vi "FL24 Washer Tool Main.vi"() -> ()   [LabVIEW 2016]
uses:
  Common/LabVIEW GEA2 Toolkit/LabVIEW_GEA2_Toolkit.lvlibp/type defs/Data In.ctl
  Common/LabVIEW GEA2 Toolkit/LabVIEW_GEA2_Toolkit.lvlibp/type defs/Source_Destination.ctl
  Common/LabVIEW GEA2 Toolkit/LabVIEW_GEA2_Toolkit.lvlibp/type defs/Data Type.ctl
  Common/LabVIEW GEA2 Toolkit/LabVIEW_GEA2_Toolkit.lvlibp/type defs/ERD Read Data In.ctl
  Laundry Tool 2.0 Support/type defs2/Select _Graph_Brass.ctl
  Laundry Tool 1.0 Support/type defs/ERD_Graph_All.ctl
  Laundry Tool 1.0 Support/type defs/ERD_Graph.ctl
  Laundry Tool 1.0 Support/type defs/Version.ctl
  Laundry Tool 2.0 Support/type defs2/ERD_Always_Show_Brass.ctl
  Laundry Tool 1.0 Support/type defs/Fault_Buffer_Status.ctl
  Laundry Tool 2.0 Support/type defs2/Diagnostics_Table.ctl
  Laundry Tool 1.0 Support/type defs/Cycle_Diag_Buffer_Status.ctl
  Laundry Tool 1.0 Support/type defs/Motor Control.ctl
  Laundry Tool 1.0 Support/type defs/Valves.ctl
  Laundry Tool 2.0 Support/type defs2/Programming_Brass.ctl
  Laundry Tool 2.0 Support/type defs2/Flash_Results.ctl
  Laundry Tool 2.0 Support/type defs2/ERD_Data_Loop_Control_Brass.ctl
  Laundry Tool 2.0 Support/type defs2/ERD_Loop_States_Brass.ctl
  Laundry Tool 2.0 Support/type defs2/Error_Command_Brass.ctl
  Laundry Tool 2.0 Support/type defs2/DAQ_States_Brass.ctl
  Common/GExplorer Support/typedefs/GExplorer_Data_Cluster.ctl
  Laundry Tool 1.0 Support/type defs/Cont_Send_States.ctl
  Laundry Tool 2.0 Support/type defs2/Cont_Send_States_Brass.ctl
  Common/LabVIEW GEA2 Toolkit/LabVIEW_GEA2_Toolkit.lvlibp/type defs/Data Out.ctl
  Common/LabVIEW GEA2 Toolkit/LabVIEW_GEA2_Toolkit.lvlibp/type defs/ERD Write Data In.ctl
  Laundry Tool 2.0 Support/type defs2/DAQ_Control_Command_Brass.ctl
  Laundry Tool 2.0 Support/type defs2/ERD_Loop_Control_Command_Brass.ctl
  Laundry Tool 2.0 Support/type defs2/GEA2_Control_Command_Brass.ctl
  <vilib>/DAQmx/read.llb/DAQmx Read (Digital 1D Bool NChan 1Samp 1Line).vi
  <vilib>/DAQmx/read.llb/DAQmx Read (Digital 1D U8 1Chan NSamp).vi
  <vilib>/DAQmx/write.llb/DAQmx Write (Digital Bool 1Line 1Point).vi
  <vilib>/DAQmx/read.llb/DAQmx Read (Counter U32 1Chan 1Samp).vi
  <vilib>/DAQmx/write.llb/DAQmx Write (Analog 1D DBL NChan 1Samp).vi
  <vilib>/DAQmx/write.llb/DAQmx Write (Digital 1D Bool NChan 1Samp 1Line).vi
  Common/LabVIEW GEA2 Toolkit/LabVIEW_GEA2_Toolkit.lvlibp/advanced/GEA2 Message Received Event Handler.vi
  <vilib>/DAQmx/create/channels.llb/DAQmx Create Channel (DO-Digital Output).vi
  <vilib>/DAQmx/create/channels.llb/DAQmx Create Channel (DI-Digital Input).vi
  <vilib>/DAQmx/configure/timing.llb/DAQmx Timing (Sample Clock).vi
  <vilib>/DAQmx/create/channels.llb/DAQmx Create Channel (CO-Pulse Generation-Frequency).vi
  <vilib>/DAQmx/configure/timing.llb/DAQmx Timing (Implicit).vi
  <vilib>/DAQmx/create/channels.llb/DAQmx Create Channel (CI-Count Edges).vi
  <vilib>/DAQmx/create/channels.llb/DAQmx Create Channel (AO-Voltage-Basic).vi
  <vilib>/DAQmx/miscellaneous.llb/DAQmx Fill In Error Info.vi
  C:/Automation/DLLs/PC Dot Net/GeaCommunication.dll
  Common/LabVIEW GEA2 Toolkit/LabVIEW_GEA2_Toolkit.lvlibp
  Automation/Product Specific/Clothes Care/2015 VA Washer/Projects/2015 VA Washer.lvlib
  <resource>/objmgr/daqmx.rc
panel:
  in  "Data ON":bool=TRUE
  out "ERD_Always Show":T1
  in  "Stop":bool
  out "Fault Status":bool
  out "Log Rate (ms)":u32
  in  "Tab Control":T2(tab)
  in  "Programming":T3={"Program"=FALSE, "File Path"=path "", "Program Ind"=FALSE, "Result"=9, "Reset Board"=FALSE, "Enter Bootloader"=FALSE} {"Result" items=["ImageRejected", "BoardNotFound", "UnableToGetGeaConfiguration", "WriteToFlashNotAllowed", "ImageDownloadedSuccessfully", "ImagePresent", "WriteToFlashFailed", "EraseFailed", "CrcFailed", ""]}
  in  "Filter Data":bool=TRUE
  in  "Start Send":bool
  in  "Cmd":string
  in  "Filter Log":bool
  in  "Msg Rate (ms)":u32=1000 min=50 step=50
  out "CSV File Log Path":path=path "C:/Users/502129737/Desktop/1"
  in  "Clear":bool
  out "GEA2 Log":string
  in  "Board Index":u8 max=0 step=1
  out "Board ID":string="0"
  in  "GEA2 Send":T5={"Source"=228, "Destination"=52, "Command"=0, "Message"=""} {"Command" format="%02x"; "Destination" format="%02x"; "Source" format="%02x"}
  in  "Send Button":bool
  in  "GEA2 Log Length":i32=100000
  in  "Save Log":bool
  out "Version":T6
  in  "GEA Inputs":T7={"Source"=228, "Destination"=52} {"Destination" format="%.0x"; "Source" format="%.0x"}
  in  "Read ERD List":T8[](array[typedef])=[{"ERD Number"=0, "Data Type"=enum."string"}] {"ERD Number" format="%.0x"}
  out "Read ERD Data Out":cluster{"ERD Number":u16, "Data":string}[](array[cluster]) {"ERD Number" format="%.0x"}
  in  "Read ERD":bool
  in  "Write ERD":bool
  in  "Write ERD List":T10(array[cluster])=[{"ERD Number"=0, "Data Type"=enum."string", "Data"=""}] {"ERD Number" format="%.0x"}
  out "All Loads":u16[][](graph)=[[0, 100, 200, 300, 400]]
  in  "ERD Graphing ON":bool
  out "ERD Graph  Ind":T11
  in  "ERD Graph Cntrl":T12={"ERD 3"={"ERD #"=61458, "Data Type"=enum."uint16_t", "Scaler"=100}, "ERD 2"={"ERD #"=61458, "Data Type"=enum."uint16_t", "Scaler"=100}, "ERD 1"={"ERD #"=61458, "Data Type"=enum."uint16_t", "Scaler"=100}} {"ERD 1"."Scaler" min=1; "ERD 1"."ERD #" format="%.0x"; "ERD 2"."Scaler" min=1; "ERD 2"."ERD #" format="%.0x"; "ERD 3"."Scaler" min=1; "ERD 3"."ERD #" format="%.0x"}
  in  "Graphing ON":bool=TRUE
  in  "Select Graph":T14
  out "ERD 3":dbl(graph)
  out "ERD 2":dbl(graph)
  out "ERD 1":dbl(graph)
  out "Water Temperature":dbl(graph)
  out "Basket Speed":u16(graph)
  out "Pressure 2":dbl(graph)
  in  "Save Fault Log":bool
  in  "Clear Fault Table Buffer":bool
  in  "Clear Fault Seq Buffer":bool
  in  "Fault ON":bool
  out "Fault Table Buffer":string[][](table)
  out "Fault Sequence Buffer":string
  out "Seq Buffer Status":T15
  out "Table Buffer Status":T15
  in  "Save Cycle History Log":bool
  in  "Clear Cycle Buffer":bool
  out "Cycle Buffer Status":T16
  in  "Get Cycle History":bool
  out "Diagnostics Table":T17
  in  "Buzzer":cluster{"Test":bool}
  in  "Drain Pump":cluster{"ON":bool, "OFF":bool}
  in  "Valve Control":T18
  in  "Motor Control":T19={"Speed (RPM)"=50, "Start Motor"=FALSE, "Stop Motor"=FALSE} {"Speed (RPM)" min=-100 max=1400 step=50}
  in  "Test Mode":cluster{"Exit":bool, "Enter":bool}
  in  "Door Lock":cluster{"Lock Door":bool, "Unlock Door":bool}
  in  "LEDs":cluster{"ON":bool, "OFF":bool}
  in  "Drum Light":cluster{"ON":bool, "OFF":bool}
  in  "Heater":cluster{"ON":bool, "OFF":bool}
  in  "HE/LE ?":enum16{"HE", "LE"}(ring)
  in  "LL (M - A)":bool=TRUE
  in  "Lid Lock Feedback":bool
  in  "MS (M - A)":bool=TRUE
  out "DAQ Status":string
  out "Drain Pump":bool
  out "Mode Shift":bool
  out "Recirc Pump":bool
  out "Cold Valve":bool
  out "Hot Valve":bool
  out "Spray/Rinse Valve":bool
  out "Fabric SoftValve":bool
  in  "AC Power":bool=TRUE
  in  "Mode Shift FB":bool
  in  "Lid Status":bool=TRUE
  in  "Pressure":dbl(slide) min=0.0 max=5.0 step=0.5 scale=0.0..5.0 scale format="%#_3g"
  in  "Motor Current":dbl(slide)=2.5 min=0.0 max=5.0 step=0.5 scale=0.0..5.0 scale format="%#_3g"
  in  "Turn On DAQ":bool
  out "DAQ On?":bool
  in  "Basket RPM":dbl=1.0 min=1.0 max=800.0 step=5.0
  in  "Temperature":dbl(slide)=2.5 min=0.0 max=5.0 step=0.5 scale=0.0..5.0 scale format="%#_3g"
  out "Triac CW":bool
  out "Traic CCW":bool
  out "CCW":u32
  out "CW":u32
  in  "ERD Read List":T20(array[cluster])=[{"Boolean"=TRUE, "ERD Number"=1, "ERD Name"="Model Number", "Data Type"=enum."string"}, {"Boolean"=TRUE, "ERD Number"=2, "ERD Name"="Serial Number", "Data Type"=enum."string"}, {"Boolean"=TRUE, "ERD Number"=8192, "ERD Name"="Machine Status", "Data Type"=enum."uint8_t"}, {"Boolean"=TRUE, "ERD Number"=8202, "ERD Name"="Cycle Name", "Data Type"=enum."string"}, {"Boolean"=TRUE, "ERD Number"=8213, "ERD Name"="Soil Level", "Data Type"=enum."string"}, {"Boolean"=TRUE, "ERD Number"=142, "ERD Name"="Cycle Count", "Data Type"=enum."uint32_t"}, {"Boolean"=TRUE, "ERD Number"=8193, "ERD Name"="Sub-Cycle", "Data Type"=enum."string"}, {"Boolean"=TRUE, "ERD Number"=141, "ERD Name"="System Runtime", "Data Type"=enum."uint32_t"}, {"Boolean"=TRUE, "ERD Number"=8208, "ERD Name"="Delay Time", "Data Type"=enum."uint16_t"}, {"Boolean"=TRUE, "ERD Number"=70, "ERD Name"="Cycle Time", "Data Type"=enum."uint16_t"}, {"Boolean"=TRUE, "ERD Number"=8206, "ERD Name"="Operating Mode", "Data Type"=enum."string"}, {"Boolean"=TRUE, "ERD Number"=8214, "ERD Name"="Temp Level", "Data Type"=enum."uint8_t"}, {"Boolean"=TRUE, "ERD Number"=8215, "ERD Name"="Spin Level", "Data Type"=enum."uint8_t"}, {"Boolean"=TRUE, "ERD Number"=61440, "ERD Name"="Water Level", "Data Type"=enum."uint8_t"}, {"Boolean"=TRUE, "ERD Number"=8216, "ERD Name"="Rinse Option", "Data Type"=enum."uint8_t"}, {"Boolean"=TRUE, "ERD Number"=4, "ERD Name"="Control Lock", "Data Type"=enum."string"}, {"Boolean"=TRUE, "ERD Number"=10, "ERD Name"="Signal Volume", "Data Type"=enum."string"}, {"Boolean"=TRUE, "ERD Number"=61457, "ERD Name"="Basket Speed", "Data Type"=enum."uint16_t"}, {"Boolean"=TRUE, "ERD Number"=8210, "ERD Name"="Door Status", "Data Type"=enum."string"}, {"Boolean"=TRUE, "ERD Number"=8211, "ERD Name"="Lock Status", "Data Type"=enum."string"}, {"Boolean"=TRUE, "ERD Number"=8258, "ERD Name"="Pressure (inches)", "Data Type"=enum."uint16_t"}, {"Boolean"=TRUE, "ERD Number"=8259, "ERD Name"="Water Temperature", "Data Type"=enum."uint16_t"}, {"Boolean"=TRUE, "ERD Number"=61458, "ERD Name"="Pressure Hz", "Data Type"=enum."uint16_t"}, {"Boolean"=TRUE, "ERD Number"=61455, "ERD Name"="Load Status 2", "Data Type"=enum."uint8_t"}, {"Boolean"=TRUE, "ERD Number"=61456, "ERD Name"="Load Status 1", "Data Type"=enum."uint8_t"}, {"Boolean"=TRUE, "ERD Number"=61460, "ERD Name"="Firmware Version", "Data Type"=enum."string"}, {"Boolean"=FALSE, "ERD Number"=61452, "ERD Name"="Drum Light", "Data Type"=enum."string"}] {"ERD Number" format="%.0x"}
  out "Error Out":errorcluster
  in  "Error In":errorcluster
  # "Software Version"
  # "UI"
  # "MC"
  # "INV"
  # "PERSONALITY"
  # "Must input a valid ERD# and Data Type\nDO NOT Leave Blank \nIf no scaler use value of 01"
  # "+ CCW   - CW"
  # "Contact:\n\nDerek Hibdon\nderek.hibdon@ge.com"
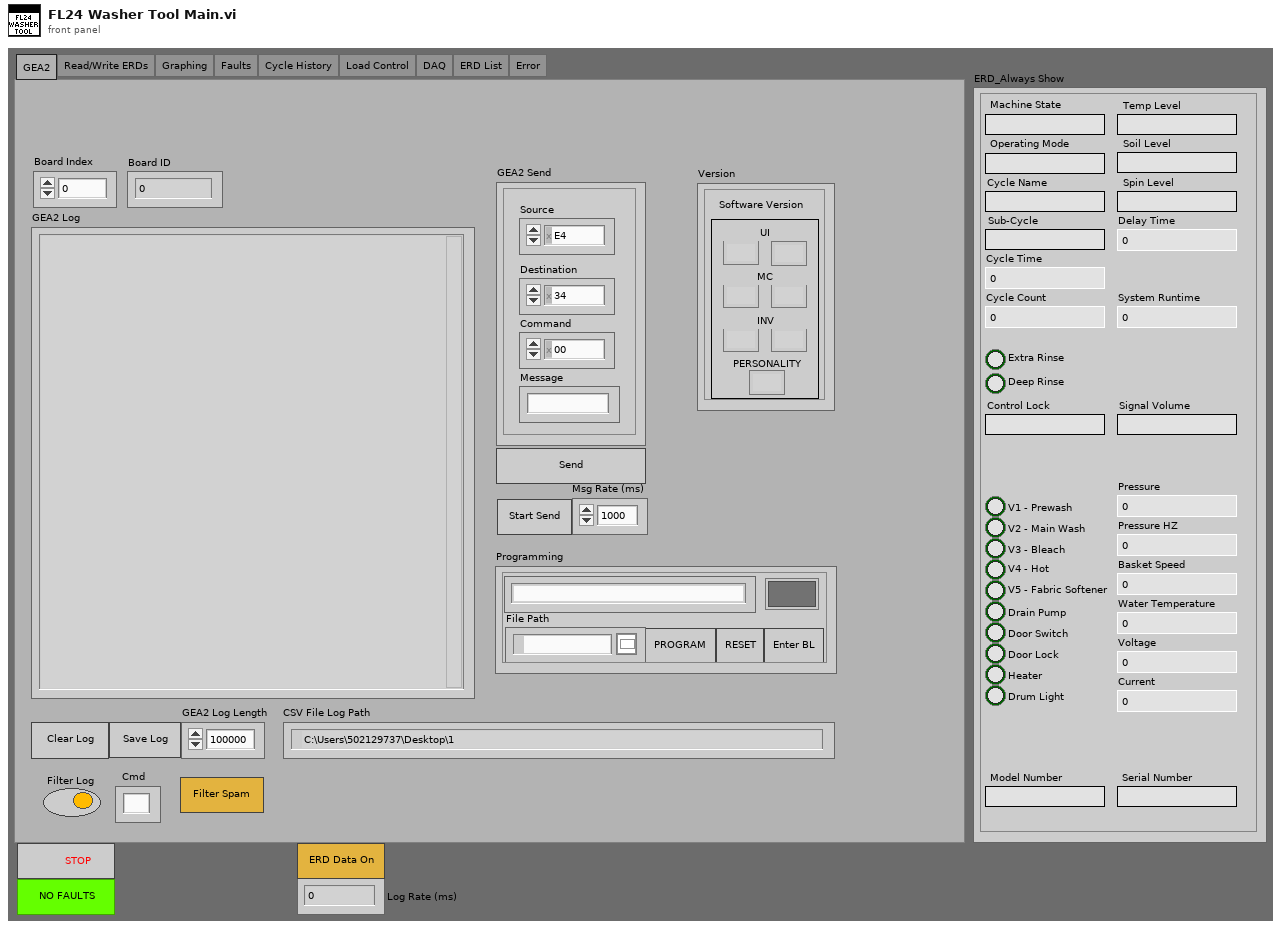
[diagram p1: front panel]
types:
  T1 = typedef "ERD_Always_Show_Brass.ctl" = cluster{"Machine State":string, "Cycle Count":u32, "Soil Level":string, "Spin Level":string, "Temp Level":string, "Delay Time":u16, "Sub-Cycle":string, "Cycle Name":string, "Model Number":string, "Serial Number":string, "System Runtime":u32, "Cycle Time":u16, "Operating Mode":string, "Deep Rinse":bool, "Extra Rinse":bool, "V1 - Prewash":bool, "V2 - Main Wash":bool, "V3 - Bleach":bool, "V4 - Hot":bool, "Drain Pump":bool, "Door Switch":bool, "Door Lock":bool, "Basket Speed":u16, "Water Temperature":dbl, "Voltage":u16, "Pressure":dbl, "Heater":bool, "Control Lock":string, "Signal Volume":string, "Current":u16, "Pressure HZ":dbl, "Drum Light":bool, "V5 - Fabric Softener":bool}
  T2 = enum32{"GEA2", "Read/Write ERDs", "Graphing", "Faults", "Cycle History", "Load Control", "DAQ", "ERD List", "Error"}
  T3 = typedef "Programming_Brass.ctl" = cluster{"Program":bool, "File Path":path, "Program Ind":bool, "Result":T4, "Reset Board":bool, "Enter Bootloader":bool}
  T4 = typedef "Flash_Results.ctl" = i32
  T5 = typedef "LabVIEW_GEA2_Toolkit.lvlibp/Data In.ctl" = cluster{"Source":u8, "Destination":u8, "Command":u8, "Message":string}
  T6 = typedef "Version.ctl" = cluster{"UI Major":string, "UI Minor":string, "MC Minor":string, "MC Major":string, "Inverter Minor":string, "Inverter Major":string, "Personality":string}
  T7 = typedef "LabVIEW_GEA2_Toolkit.lvlibp/Source_Destination.ctl" = cluster{"Source":u8, "Destination":u8}
  T8 = typedef "LabVIEW_GEA2_Toolkit.lvlibp/ERD Read Data In.ctl" = cluster{"ERD Number":u16, "Data Type":T9}
  T9 = typedef "LabVIEW_GEA2_Toolkit.lvlibp/Data Type.ctl" = enum16{"string", "boolean", "uint8_t", "uint16_t", "uint32_t", "uint64_t", "int8_t", "int16_t", "int32_t", "int64_t"}
  T10 = cluster{"ERD Number":u16, "Data Type":T9, "Data":string}[]
  T11 = cluster{"ERD Value 1":dbl, "ERD Value 2":dbl, "ERD Value 3":dbl}
  T12 = typedef "ERD_Graph_All.ctl" = cluster{"ERD 3":T13, "ERD 2":T13, "ERD 1":T13}
  T13 = typedef "ERD_Graph.ctl" = cluster{"ERD #":u16, "Data Type":T9, "Scaler":u32}
  T14 = typedef "Select _Graph_Brass.ctl" = enum16{"All Loads", "ERD 1", "ERD 2", "ERD 3", "Temperature (F)", "Basket Speed (RPM)", "Pressure (in H2O)"}
  T15 = typedef "Fault_Buffer_Status.ctl" = cluster{"Current Index":u16, "Count":u16, "Overwrite Count":u16}
  T16 = typedef "Cycle_Diag_Buffer_Status.ctl" = cluster{"Current Index":u16, "Count":u16, "Overwrite Count":u16}
  T17 = typedef "Diagnostics_Table.ctl" = string[][]
  T18 = typedef "Valves.ctl" = cluster{"PreWash Valve":bool, "Bleach Valve":bool, "Hot Valve":bool, "Valves ON":bool, "Valves OFF":bool, "MainWash Valve":bool, "Fabric Softener":bool}
  T19 = typedef "Motor Control.ctl" = cluster{"Speed (RPM)":i16, "Start Motor":bool, "Stop Motor":bool}
  T20 = cluster{"Boolean":bool, "ERD Number":u16, "ERD Name":string, "Data Type":enum16{"string", "boolean", "uint8_t", "uint16_t", "uint32_t", "uint64_t"}}[]
  T21 = typedef "Cont_Send_States_Brass.ctl" = enum16{"Run", "Shutdown"}
  T22 = typedef "Cont_Send_States.ctl" = enum16{"Run", "Shutdown"}
  T23 = typedef "GExplorer_Data_Cluster.ctl" = cluster{"Data":variant, "State":enum16{"Add to Log", "Clear", "Shutdown"}}
  T24 = typedef "DAQ_States_Brass.ctl" = enum16{"Wait for Init", "Rename Devices", "Verify Hardware", "Initialize", "Run", "Shutdown", "Exit"}
  T25 = typedef "ERD_Data_Loop_Control_Brass.ctl" = cluster{"Data":variant, "State":T26}
  T26 = typedef "ERD_Loop_States_Brass.ctl" = enum16{"Init", "Build ERD Read List", "Read ERDs", "Update UI", "Update Graphs", "Read Faults", "Log Data", "Pause", "Shutdown"}
  T27 = typedef "Error_Command_Brass.ctl" = enum16{"Initialize", "Handle Errors", "Report Errors"}
  T28 = typedef "LabVIEW_GEA2_Toolkit.lvlibp/ERD Write Data In.ctl" = cluster{"ERD Number":u16, "Data Type":T9, "Data":string}
  T29 = enum8{"Enabled", "Disabled", "Disabled and Grayed Out"}
  T30 = typedef "GEA2_Control_Command_Brass.ctl" = enum16{"Initialize", "Shutdown"}
  T31 = typedef "ERD_Loop_Control_Command_Brass.ctl" = enum16{"Initialize", "Shutdown"}
  T32 = typedef "DAQ_Control_Command_Brass.ctl" = enum16{"Initialize", "Shutdown", "Exit"}
  T33 = typedef "LabVIEW_GEA2_Toolkit.lvlibp/Data Out.ctl" = cluster{"Source":u8, "Destination":u8, "Command":u8, "Length":u8, "CRC":u16, "Message":string}
  T34 = typedef "LabVIEW_GEA2_Toolkit.lvlibp/ERD Read Data Out.ctl" = cluster{"ERD Number":u16, "Data":string}
  T35 = typedef "All_Bundled_Data_Brass.ctl" = cluster{"Version":T6, "ERD_Always Show":T1, "Personality Set":u8, "CSV File String Arrays":T36, "Fault Table Array ":T37}
  T36 = typedef "CSV_File_String_Arrays.ctl" = cluster{"ERD Number Array":string[], "ERD Name Array":string[], "ERD Converted String Data":string[]}
  T37 = typedef "Fault Table Array.ctl" = T38[]
  T38 = typedef "Fault_Table_Info.ctl" = cluster{"Cycle Count":u32, " Runtime (min) ":u32, "Fault Status":string, "Fault ID":string, "Fault Count":u16}
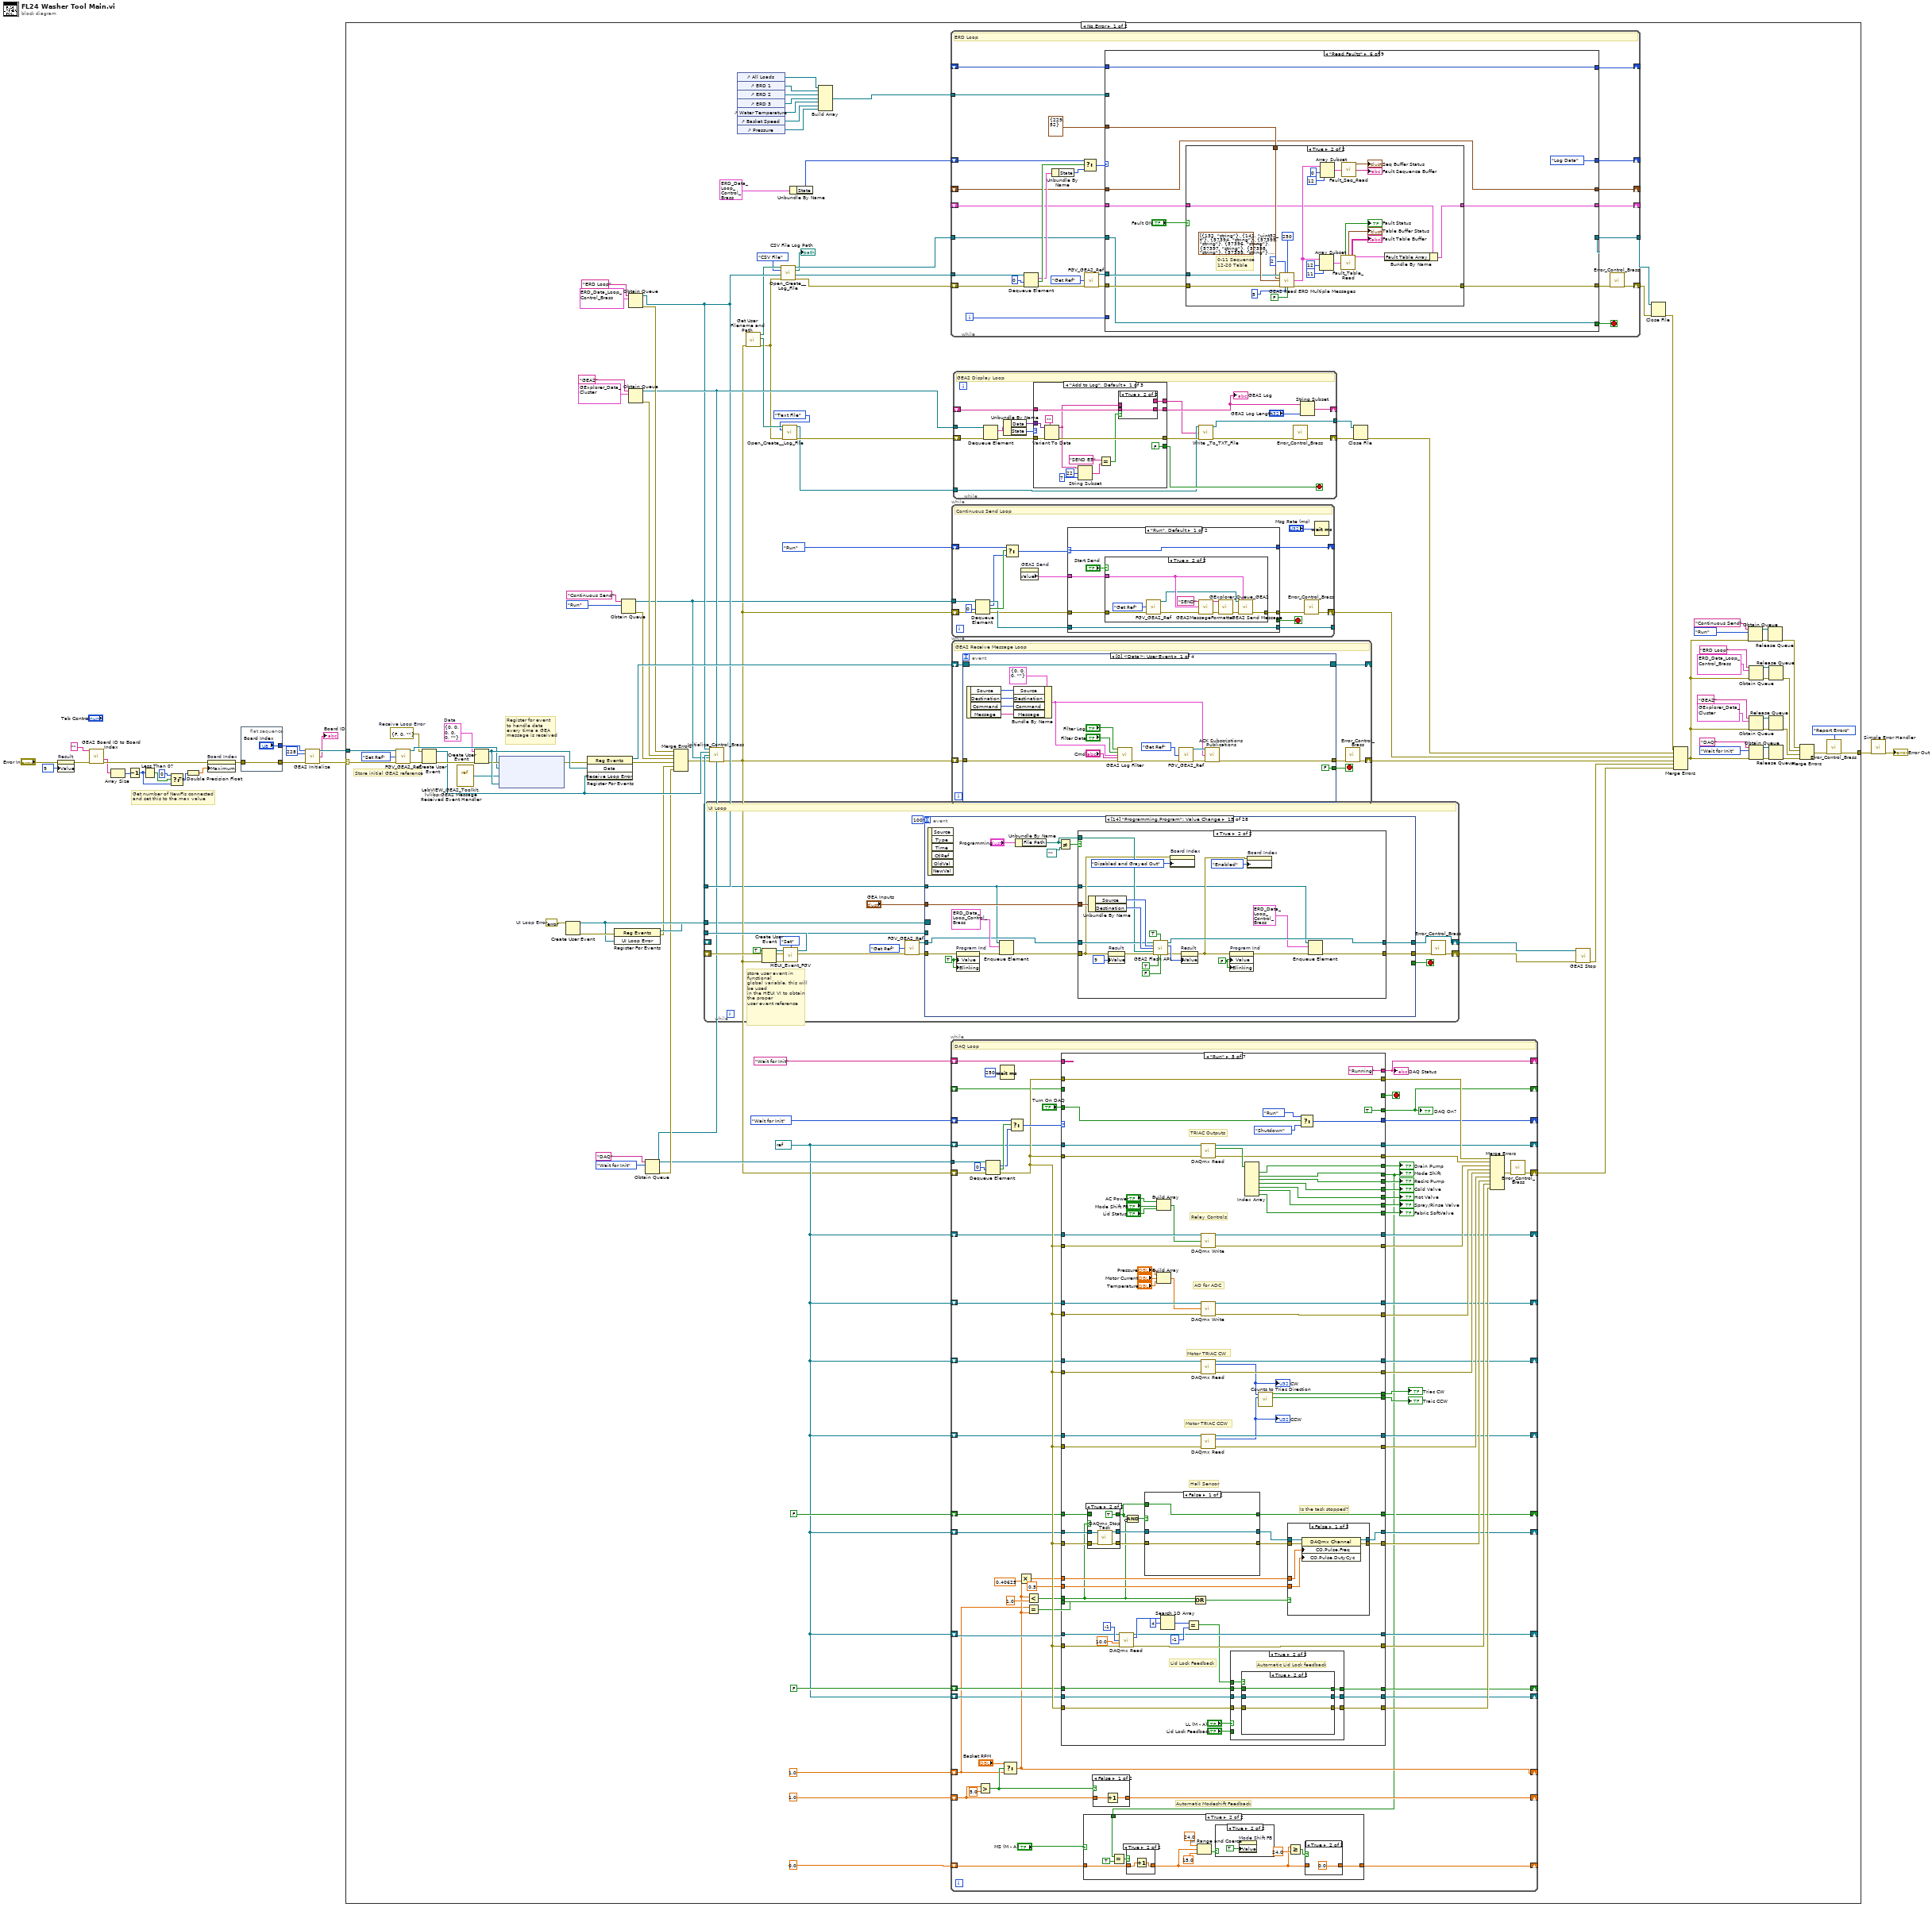
[diagram p0: block diagram]
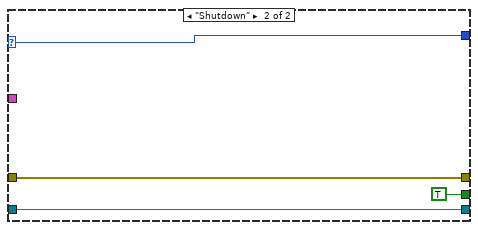
[diagram p3: hidden frame]
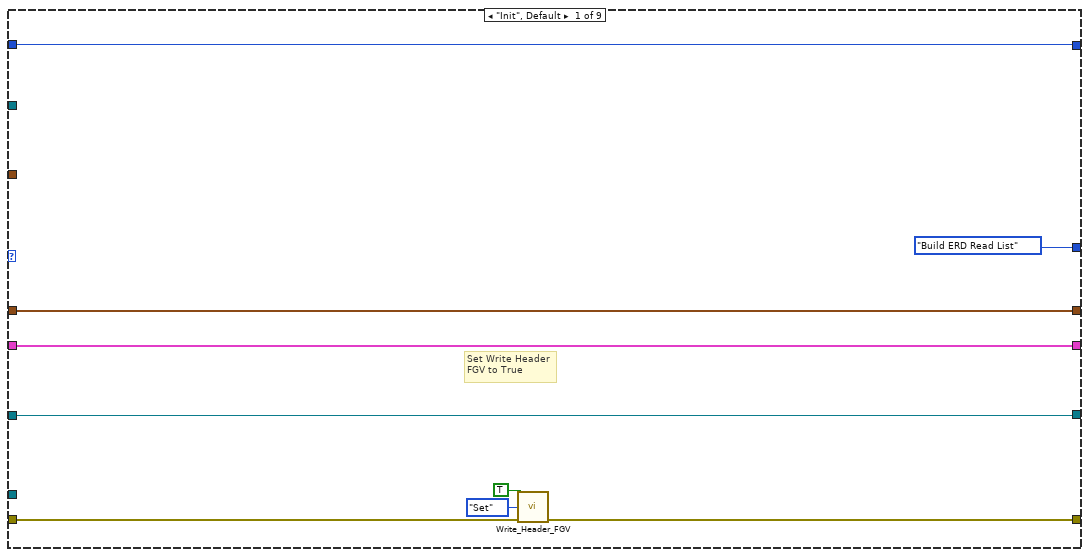
[diagram p4: hidden frame]
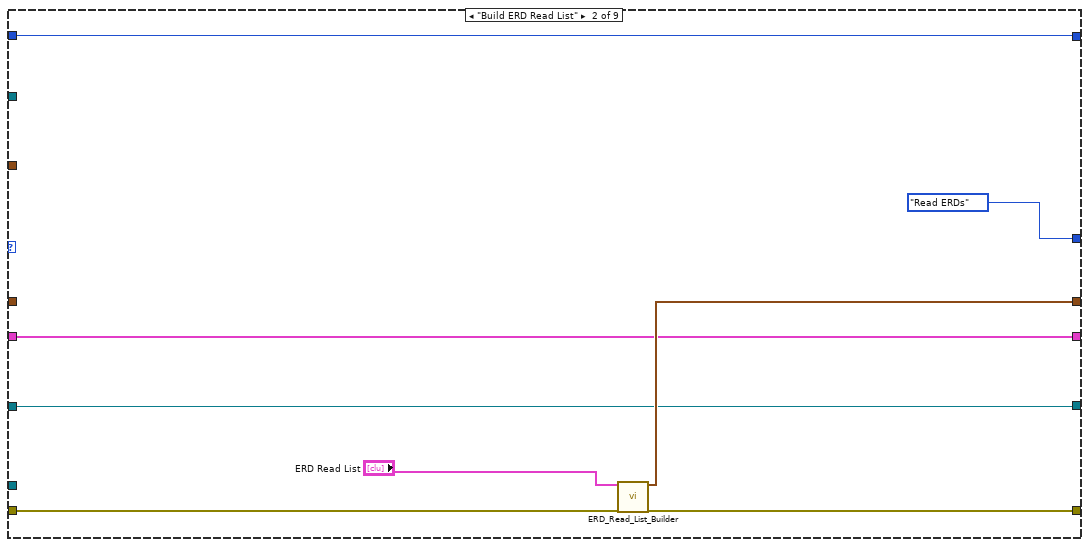
[diagram p5: hidden frame]
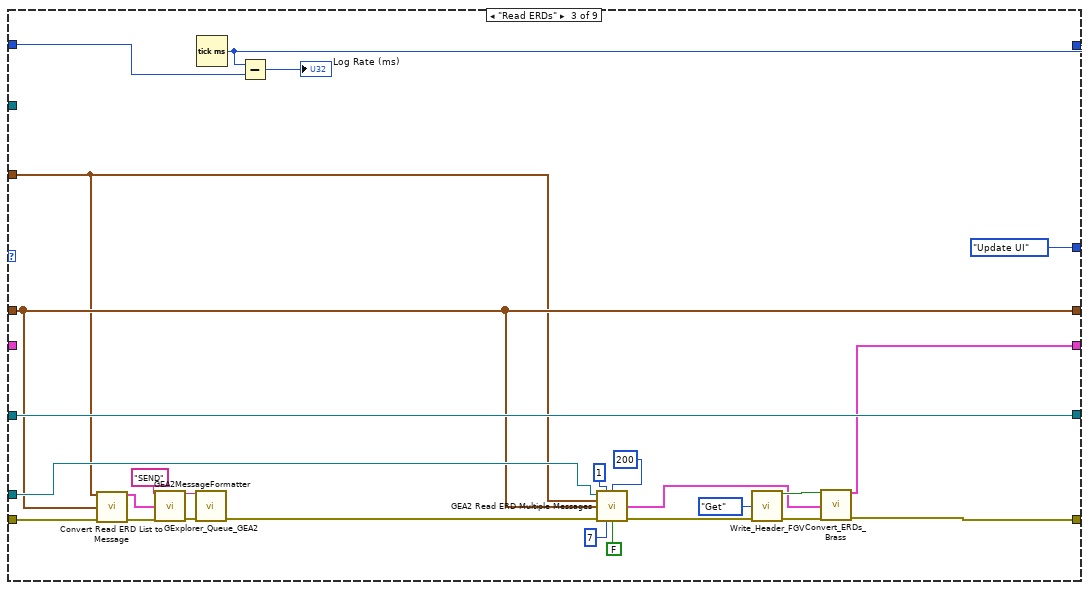
[diagram p6: hidden frame]
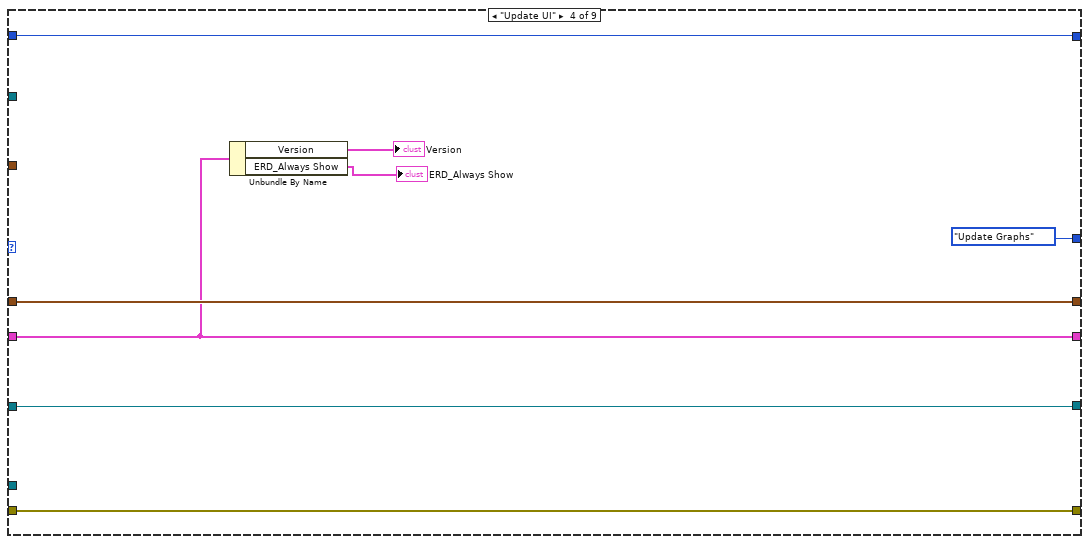
[diagram p7: hidden frame]
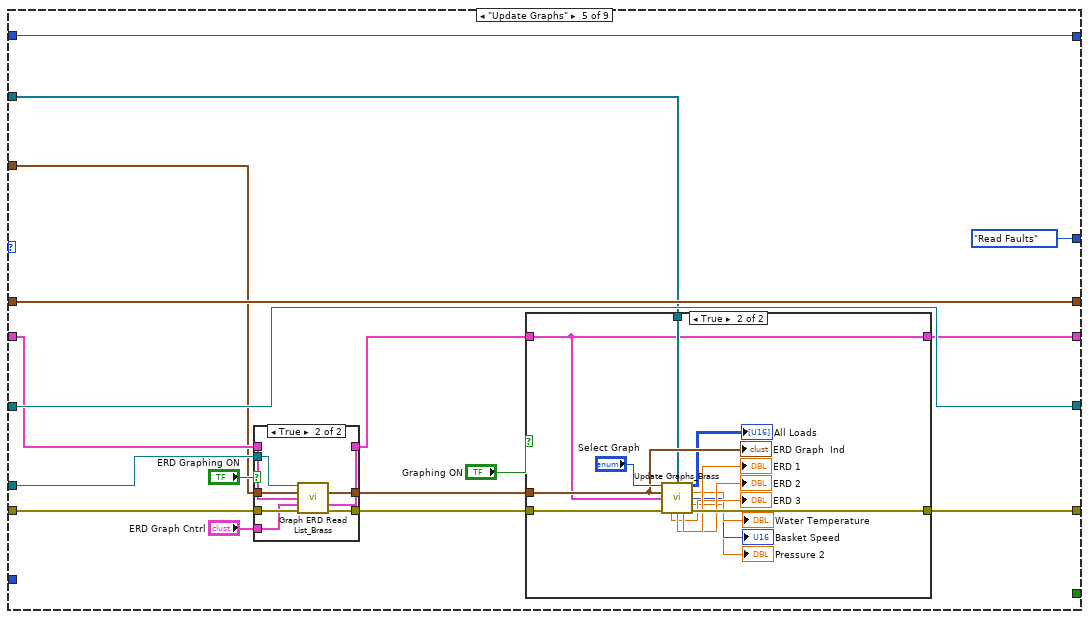
[diagram p8: hidden frame]
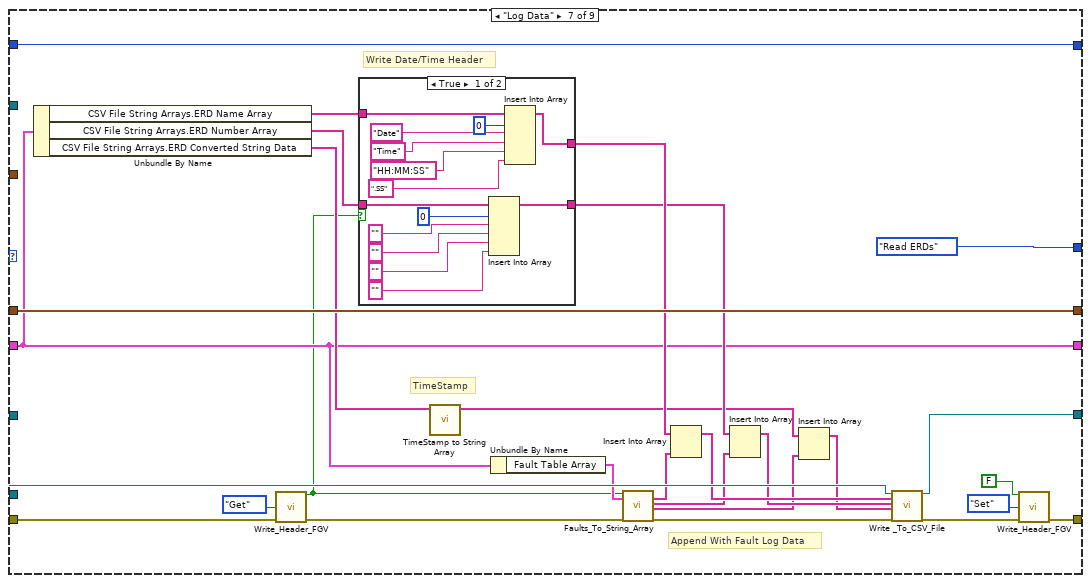
[diagram p12: hidden frame]
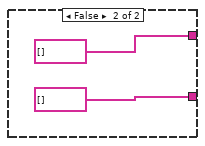
[diagram p13: hidden frame]
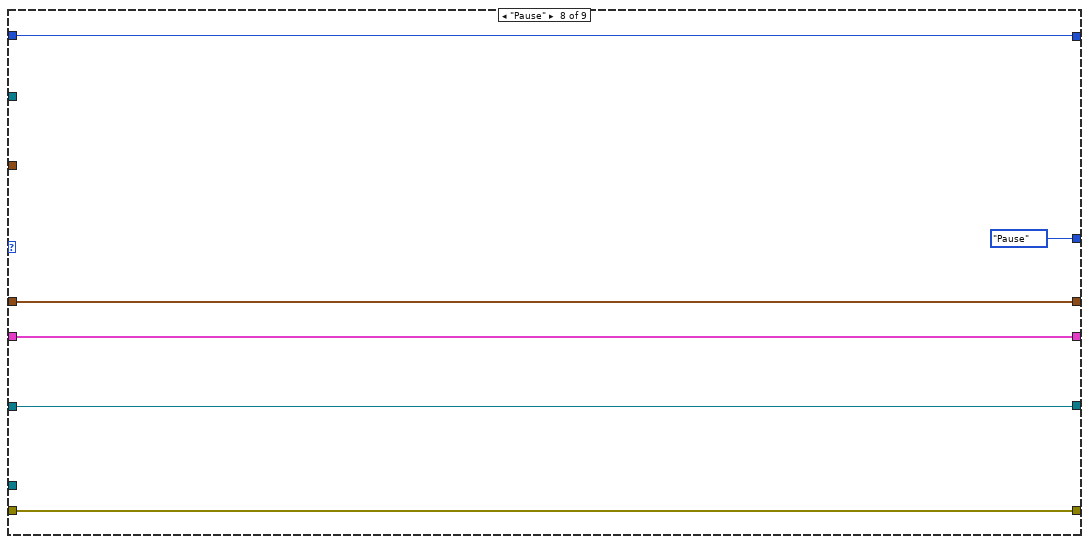
[diagram p14: hidden frame]
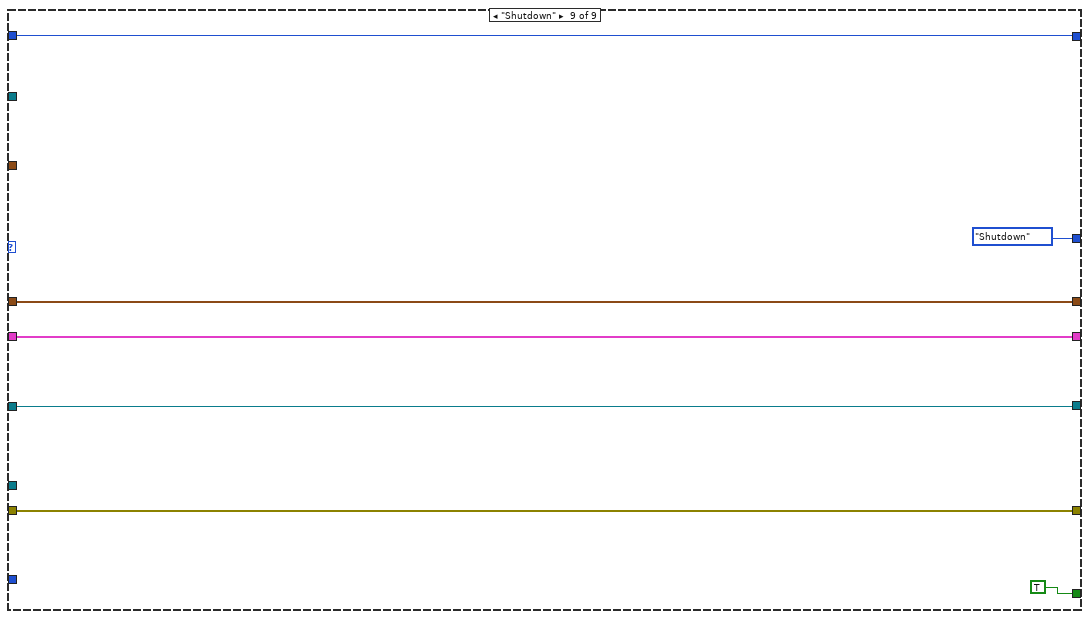
[diagram p15: hidden frame]
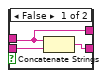
[diagram p16: hidden frame]
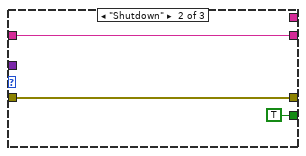
[diagram p17: hidden frame]
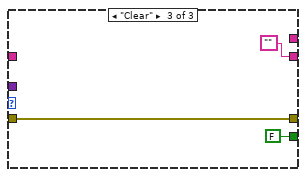
[diagram p18: hidden frame]
diagram:
  w1 = T4 9 items=["ImageRejected", "BoardNotFound", "UnableToGetGeaConfiguration", "WriteToFlashNotAllowed", "ImageDownloadedSuccessfully", "ImagePresent", "WriteToFlashFailed", "EraseFailed", "CrcFailed", ""] ("Value")
  # "Get number of NewFIs connected\nand set this to the max value"
  n1 = property on="Result" class="Ring (strict)"(error in="Error In", "Value"=w1) -> (error out=w2:errorcluster)  [unwired: 1 in, 1 out]
  n2 = call "GEA2 Board ID to Board Index.vi"("Board ID"="", "Error In"=w2) -> ("Boards Found"=w7:string[], "Error Out"=w15:errorcluster)  [unwired: 9 in, 3 out]
  n3 = Array Size(array=w7) -> (size(s)=w12:i32)
  n4 = Decrement(x=w12) -> (x-1=w10:i32)
  n5 = Less Than 0?(x=w10) -> (x < 0?=w11:bool)
  n6 = Select(t=0, s=w11, f=w10) -> (s? t:f=w8:i32)
  n7 = To Double Precision Float(number=w8) -> (double precision float=w6:dbl)
  n8 = property on="Board Index" class="DigNum (strict)"(error in=w15, "Maximum"=w6) -> (error out=w14:errorcluster)  [unwired: 1 in, 1 out]
  n9 = flat-sequence {
    tunnel: ["Board Index"] -> w18
    tunnel: w14 -> [w22]
    tunnel: [w22] -> w13
    frame #0 {
    }
  }
  n10 = call "GEA2 Initialize.vi"("Board Index"=w18, "Source Address"=u8 228, "error in"=w13) -> ("GEA2 Reference Out"=w20:refnum<k24>, "Board ID"=→"Board ID":string, "error out"=w19:errorcluster)  [unwired: 10 in]
  n11 = case shown="No Error" w19 {
    selector: w19 -> [w86 w1782]
    tunnel: w20 -> [w84 _]
    tunnel: [w88 w1782] -> w5
    frame No Error {
      w40 = errorcluster {"status"=FALSE, "code"=0, "source"=""}  # Receive Loop Error
      w41 = T33 {"Source"=0, "Destination"=0, "Command"=0, "Length"=0, "CRC"=0, "Message"=""}  # Data
      w56 = refnum<k21> refnum ("task out")
      w122 = errorcluster {"status"=FALSE, "code"=0, "source"=""}  # UI Loop Error
      # "store user event in functional\nglobal variable, this will be used\nin the HEUI VI to obtain the proper\nuser event reference"
      # "Store initial GEA2 reference"
      # "Register for event\nto handle data\nevery time a GEA\nmessage is received"
      n12 = call "FGV_GEA2_Ref.vi"("GEA2 Reference In"=w84, "Action"=enum16{"Set Ref", "Get Ref"}."Set Ref", "Error In"=w86) -> ("GEA2 Reference Out"=w83:refnum<k24>, "Error Out"=w85:errorcluster)  [unwired: 11 in]
      n13 = Create User Event(user event datatype=w40, error in=w85) -> (user event=w123:refnum<user-event>, error out=w125:errorcluster)
      n14 = vi-ref "LabVIEW_GEA2_Toolkit.lvlibp:GEA2 Message Received Event Handler.vi"() -> (w124:refnum<vi>)
      n15 = Create User Event(user event datatype=w41, error in=w125) -> (user event=w128:refnum<user-event>, error out=w127:errorcluster)
      n16 = node(w127, w83, w124, w128) -> (w126:errorcluster)  [unwired: 1 in, 1 out]
      n17 = Create User Event(user event datatype=w122) -> (user event=w111:refnum<user-event>, error out=w121:errorcluster)  [unwired: 1 in]
      n18 = register-events(error in=w126, w128, w123) -> (reference out=w120:refnum<event-registration>, error out=w93:errorcluster)  [unwired: 1 in]
      n19 = register-events(error in=w121, w111) -> (reference out=w102:refnum<event-registration>, error out=w92:errorcluster)  [unwired: 1 in]
      n20 = Obtain Queue(name (unnamed)="Continuous Send", element data type=Cont_Send_States_Brass."Run" ("State")) -> (queue out=w42:refnum<queue>, error out=w47:errorcluster)  [unwired: 3 in, 1 out]
      n21 = Obtain Queue(name (unnamed)="ERD Loop", element data type=T25 {"Data"=variant, "State"=enum."Read ERDs"} ("Data")) -> (queue out=w71:refnum<queue>, error out=w89:errorcluster)  [unwired: 3 in, 1 out]
      n22 = Obtain Queue(name (unnamed)="GEA2", element data type=T23 {"Data"=variant, "State"=enum."Add to Log"} ("Data")) -> (queue out=w72:refnum<queue>, error out=w94:errorcluster)  [unwired: 3 in, 1 out]
      n23 = Obtain Queue(name (unnamed)="DAQ", element data type=DAQ_States_Brass."Wait for Init" ("States")) -> (queue out=w64:refnum<queue>, error out=w91:errorcluster)  [unwired: 3 in, 1 out]
      n24 = Merge Errors(w89, w94, w47, w93, w92, w91) -> (w90:errorcluster)
      n25 = call "Initialize_Control_Brass.vi"("ERD Loop"=w71, "GEA2"=w72, "Receive Loop"=w123, "UI Loop Error"=w111, "Cont Send"=w42, "Error In"=w90, "DAQ"=w64) -> ("Error Out"=w37:errorcluster)  [unwired: 8 in]
      n26 = control-ref of="All Loads"() -> (w27:refnum<vi>)
      n27 = control-ref of="ERD 1"() -> (w68:refnum<vi>)
      n28 = control-ref of="ERD 2"() -> (w66:refnum<vi>)
      n29 = control-ref of="ERD 3"() -> (w67:refnum<vi>)
      n30 = control-ref of="Water Temperature"() -> (w26:refnum<vi>)
      n31 = control-ref of="Basket Speed"() -> (w25:refnum<vi>)
      n32 = control-ref of="Pressure"() -> (w24:refnum<vi>)
      n33 = call "Get User Filename and Path.vi"("error in (no error)"=w37) -> ("error out"=w29:errorcluster, "TXT File Path"=w35:path, "CSV File Path"=w38:path)  [unwired: 8 in]
      n34 = Create User Event(user event datatype=TRUE ("Bool"), error in=w37) -> (user event=w78:refnum<user-event>, error out=w79:errorcluster)
      n35 = call "Open_Create__Log_File.vi"("File Path Control"=w38, "Enum"=enum16{"CSV File", "Text File"}."CSV File", "Error In"=w29) -> ("refnum out"=w69:refnum<file>, "File Path"=→"CSV File Log Path":path, "Error Out"=w81:errorcluster)  [unwired: 10 in]
      n36 = call "Open_Create__Log_File.vi"("File Path Control"=w35, "Enum"=enum16{"CSV File", "Text File"}."Text File", "Error In"=w29) -> ("refnum out"=w34:refnum<file>, "Error Out"=w36:errorcluster)  [unwired: 10 in, 1 out]
      n37 = call "HEUI_Event_FGV.vi"("Event In"=w78, "Action"=enum16{"Get", "Set"}."Set", "Error In"=w79) -> ("Event Out"=w75:refnum<user-event>, "Error Out"=w76:errorcluster)  [unwired: 11 in]
      n38 = while "UI Loop" {
        shift-right: [w1022] -> w130
        shift-left: w76 -> [w1016]
        shift-right: [w1024] -> w129
        shift-left: _ -> [_]
        tunnel: w102 -> [w1023]
        tunnel: w75 -> [w1013]
        tunnel: w71 -> [w1012]
        stop <- w1021 stop-if-true
        # "UI Loop"
        n39 = call "FGV_GEA2_Ref.vi"("Action"=enum16{"Set Ref", "Get Ref"}."Get Ref", "Error In"=w1016) -> ("GEA2 Reference Out"=w1015:refnum<k24>, "Error Out"=w1017:errorcluster)  [unwired: 12 in]
        n40 = event shown="[14] \"Programming.Program\": Value Change" {
          selector: w1023 -> [_ _ _ _ _ _ _ _ _ _ _ _ _ _ _ _ _ _ _ _ _ _ _ _ _ _ _ _]
          dyn-events: _ -> [_ _ _ _ _ _ _ _ _ _ _ _ _ _ _ _ _ _ _ _ _ _ _ _ _ _ _ _]
          timeout: 100 -> [_ _ _ _ _ _ _ _ _ _ _ _ _ _ _ _ _ _ _ _ _ _ _ _ _ _ _ _]
          tunnel: [w1030 w1040 w1041 w1047 w1061 w1071 w1084 w1091 w1094 w1113 w1128 w1172 w1216 w1262 w1339 w1378 w1417 w1431 w1475 w1519 w1546 w1590 w1640 w1659 w1673 w1691 w1711 w1722] -> w1020
          tunnel: w1017 -> [w1027 w1037 w1041 w1043 w1058 w1075 w1082 w1089 w1098 w1116 w1132 w1176 w1220 w1266 w1351 w1396 w1425 w1435 w1479 w1523 w1550 w1595 w1643 w1665 w1681 w1697 w1712 w1729]
          tunnel: [_ _ _ _ _ _ _ _ _ _ _ _ _ _ _ _ _ _ _ _ _ _ _ _ _ _ _ TRUE] -> w1021
          tunnel: w1015 -> [w1025 w1039 w1042 w1045 w1059 _ _ _ w1100 w1115 w1131 w1175 w1219 w1265 w1342 w1395 w1424 w1434 w1478 w1522 w1549 w1594 w1642 w1664 w1675 w1696 _ w1732]
          tunnel: [w1032 w1039 w1042 w1048 w1060 _ _ _ _ w1114 _ _ _ _ w1341 _ _ _ _ _ _ _ w1641 _ _ _ _ w1732] -> w1024
          tunnel: "GEA Inputs" -> [_ _ _ w1046 w1056 _ _ _ w1099 w1117 w1130 w1174 w1218 w1264 w1343 w1391 w1422 w1433 w1477 w1521 w1548 w1593 w1644 w1662 w1674 w1698 _ _]
          tunnel: w1013 -> [_ _ _ _ _ _ _ _ _ _ _ _ _ _ _ _ _ _ _ _ _ _ _ _ _ _ _ _]
          tunnel: w1012 -> [_ _ _ _ _ _ w1080 w1087 _ _ _ _ _ _ w1338 _ w1415 _ _ _ _ _ _ _ _ _ w1709 _]
          event "Send Button": Value Change {
            n41 = event-data() -> ()  [unwired: 1 in, 1 out]
            n42 = call "GEA2MessageFormatter.vi"("Prefix(Send/Recv)"="SEND", "GEA2 Data In"="GEA2 Send", "Error In"=w1027) -> ("Output String"=w1029:string, "Error Out"=w1028:errorcluster)  [unwired: 11 in]
            n43 = call "GExplorer_Queue_GEA2.vi"("Output String"=w1029, "error in (no error)"=w1028) -> ("error out"=w1031:errorcluster)  [unwired: 13 in]
            n44 = call "GEA2 Send Message.vi"("GEA2 Reference In"=w1025, "Input Data"="GEA2 Send", "Error In"=w1031) -> ("GEA2 Reference Out"=w1032:refnum<k24>, "Error Out"=w1030:errorcluster)  [unwired: 11 in]
          }
          event "Clear": Value Change {
            w1034 = T23 {"Data"=variant, "State"=enum."Clear"} ("element")
            n45 = event-data() -> ()  [unwired: 1 in, 6 out]
            n46 = Obtain Queue(name (unnamed)="GEA2", element data type=w1034, error in (no error)=w1037) -> (queue out=w1035:refnum<queue>, error out=w1038:errorcluster)  [unwired: 2 in, 1 out]
            n47 = Enqueue Element(queue=w1035, element=w1034, error in (no error)=w1038) -> (error out=w1040:errorcluster)  [unwired: 1 in, 2 out]
          }
          event Timeout {
            # "Must have timeout case to give GEA2 FGV a chance to update\nthe GEA2 reference. Otherwise, when we receive an event it may\nbe using a reference that is no longer valid."
            n48 = event-data() -> ()  [unwired: 1 in, 3 out]
          }
          event "Write ERD": Value Change {
            n49 = event-data() -> ()  [unwired: 1 in, 1 out]
            n50 = call "Convert Write ERD List to Message.vi"("GEA Inputs"=w1046, "Write ERD List"="Write ERD List", "Error In"=w1043) -> ("GEA Message"=w1052:T5, "Error Out"=w1053:errorcluster)  [unwired: 11 in]
            n51 = call "GEA2MessageFormatter.vi"("Prefix(Send/Recv)"="SEND", "GEA2 Data In"=w1052, "Error In"=w1053) -> ("Output String"=w1054:string, "Error Out"=w1055:errorcluster)  [unwired: 11 in]
            n52 = call "GExplorer_Queue_GEA2.vi"("Output String"=w1054, "error in (no error)"=w1055) -> ("error out"=w1050:errorcluster)  [unwired: 13 in]
            n53 = call "GEA2 Write ERD.vi"("GEA2 Reference In"=w1045, "GEA Inputs"=w1046, "Write ERD List"="Write ERD List", "Error In"=w1050, "Verify ERD Response?"=FALSE) -> ("GEA2 Reference Out"=w1048:refnum<k24>, "Error Out"=w1047:errorcluster)  [unwired: 8 in, 1 out]
          }
          event "Read ERD": Value Change {
            n54 = event-data() -> ()  [unwired: 1 in, 6 out]
            n55 = call "Convert Read ERD List to Message.vi"("GEA Inputs"=w1056, "Read ERD List"="Read ERD List", "Error In"=w1058) -> ("GEA Message"=w1066:T5, "Error Out"=w1057:errorcluster)  [unwired: 11 in]
            n56 = call "GEA2MessageFormatter.vi"("Prefix(Send/Recv)"="SEND", "GEA2 Data In"=w1066, "Error In"=w1057) -> ("Output String"=w1064:string, "Error Out"=w1063:errorcluster)  [unwired: 11 in]
            n57 = call "GExplorer_Queue_GEA2.vi"("Output String"=w1064, "error in (no error)"=w1063) -> ("error out"=w1067:errorcluster)  [unwired: 13 in]
            n58 = call "GEA2 Read ERD.vi"("GEA2 Reference In"=w1059, "GEA Inputs"=w1056, "Read ERD List"="Read ERD List", "Error In"=w1067, "Verify ERD Response?"=FALSE) -> ("GEA2 Reference Out"=w1060:refnum<k24>, "ERD Data Out"=→"Read ERD Data Out":T34[], "Error Out"=w1061:errorcluster)  [unwired: 7 in, 1 out]
          }
          event "Save Log": Value Change {
            n59 = event-data() -> ()  [unwired: 1 in, 6 out]
            n60 = property on="GEA2 Log" class="Str"(error in=w1075) -> (error out=w1077:errorcluster, "Value"=w1076:string)  [unwired: 1 in, 1 out]
            n61 = Write to Text File(prompt (Choose or enter file path)="Choose filename and path to save txt file to ", text=w1076, error in=w1077) -> (refnum out=w1074:refnum<file>, error out=w1073:errorcluster)  [unwired: 1 in, 1 out]
            n62 = Close File(refnum=w1074, error in=w1073) -> (error out=w1072:errorcluster)  [unwired: 1 out]
            n63 = call <vilib>:"Clear Errors.vi"("error in (no error)"=w1072, "specific error code to clear (0: all)"=43) -> ("error out"=w1071:errorcluster)  [unwired: 4 in, 1 out]
          }
          event "ERD Read List": Value Change {
            n64 = event-data() -> ()  [unwired: 1 in, 6 out]
            n65 = Enqueue Element(queue=w1080, element=T25 {"Data"=variant, "State"=enum."Build ERD Read List"}, error in (no error)=w1082) -> (error out=w1081:errorcluster)  [unwired: 1 in, 2 out]
            n66 = call "Write_Header_FGV.vi"("Write Header ? In"=TRUE, "Action"=enum16{"Get", "Set"}."Set", "Error In"=w1081) -> ("Error Out"=w1084:errorcluster)  [unwired: 11 in, 1 out]
          }
          event "Fault ON", "ERD Graphing ON": Value Change {
            n67 = event-data() -> ()  [unwired: 1 in, 6 out]
            n68 = Enqueue Element(queue=w1087, element=T25 {"Data"=variant, "State"=enum."Build ERD Read List"}, error in (no error)=w1089) -> (error out=w1088:errorcluster)  [unwired: 1 in, 2 out]
            n69 = call "Write_Header_FGV.vi"("Write Header ? In"=TRUE, "Action"=enum16{"Get", "Set"}."Set", "Error In"=w1088) -> ("Error Out"=w1091:errorcluster)  [unwired: 11 in, 1 out]
          }
          event "Save Fault Log": Value Change {
            # "0-16 Sequence\n17-27 Table"
            n70 = event-data() -> ()  [unwired: 1 in, 6 out]
            n71 = call "GEA2 Read ERD Multiple Messages.vi"("GEA2 Reference In"=w1100, "Read Timeout (ms)"=u32 250, "GEA Inputs"=w1099, "Read ERD List"=T8[] [{"ERD Number"=132, "Data Type"=enum."string"}, {"ERD Number"=141, "Data Type"=enum."uint32_t"}, {"ERD Number"=57394, "Data Type"=enum."string"}, {"ERD Number"=57395, "Data Type"=enum."string"}, {"ERD Number"=57396, "Data Type"=enum."string"}, {"ERD Number"=57397, "Data Type"=enum."string"}, {"ERD Number"=57398, "Data Type"=enum."string"}, {"ERD Number"=57399, "Data Type"=enum."string"}, {"ERD Number"=57400, "Data Type"=enum."string"}, {"ERD Number"=57401, "Data Type"=enum."string"}, {"ERD Number"=57402, "Data Type"=enum."string"}, {"ERD Number"=57403, "Data Type"=enum."string"}, {"ERD Number"=57404, "Data Type"=enum."string"}, {"ERD Number"=57405, "Data Type"=enum."string"}, {"ERD Number"=57406, "Data Type"=enum."string"}, {"ERD Number"=57407, "Data Type"=enum."string"}, {"ERD Number"=57408, "Data Type"=enum."string"}, {"ERD Number"=129, "Data Type"=enum."string"}, {"ERD Number"=57444, "Data Type"=enum."string"}, {"ERD Number"=57445, "Data Type"=enum."string"}, {"ERD Number"=57446, "Data Type"=enum."string"}, {"ERD Number"=57447, "Data Type"=enum."string"}, {"ERD Number"=57448, "Data Type"=enum."string"}, {"ERD Number"=57449, "Data Type"=enum."string"}, {"ERD Number"=57450, "Data Type"=enum."string"}, {"ERD Number"=57451, "Data Type"=enum."string"}, {"ERD Number"=57452, "Data Type"=enum."string"}, {"ERD Number"=57453, "Data Type"=enum."string"}], "Error In"=w1098, "#ERDs per message"=14 ("#ERDs per message 2"), "Verify ERD Response?"=FALSE) -> ("ERD Data Out"=w1103:T34[], "Error Out"=w1095:errorcluster)  [unwired: 5 in, 2 out]
            n72 = Array Subset(array=w1103, index=17, length=10) -> (w1104:T34[])
            n73 = Array Subset(array=w1103, index=0, length=17) -> (w1102:T34[])
            n74 = call "Fault_Seq_Read.vi"("Seq ERD In"=w1102) -> ("String"=w1097:string)  [unwired: 13 in, 1 out]
            n75 = call "Fault_Table_Read.vi"("ERD Data Out"=w1104) -> ("Fault Table String Out"=w1096:string[][])  [unwired: 11 in, 3 out]
            n76 = call "Fault_Logging.vi"("String"=w1097, "Fault Table String Out"=w1096, "error in (no error)"=w1095) -> ("error out"=w1094:errorcluster)  [unwired: 12 in]
          }
          event "Clear Fault Seq Buffer": Value Change {
            n77 = event-data() -> ()  [unwired: 1 in, 6 out]
            n78 = Bundle By Name(cluster=T28 {"ERD Number"=133, "Data Type"=enum."string", "Data"=""} ("ERD Read Data In"), "Data"="FF") -> (w1126:T28)
            n79 = Build Array(w1126) -> (w1120:T28[])
            n80 = call "Convert Write ERD List to Message.vi"("GEA Inputs"=w1117, "Write ERD List"=w1120, "Error In"=w1116) -> ("GEA Message"=w1122:T5, "Error Out"=w1123:errorcluster)  [unwired: 11 in]
            n81 = call "GEA2MessageFormatter.vi"("Prefix(Send/Recv)"="SEND", "GEA2 Data In"=w1122, "Error In"=w1123) -> ("Output String"=w1124:string, "Error Out"=w1125:errorcluster)  [unwired: 11 in]
            n82 = call "GExplorer_Queue_GEA2.vi"("Output String"=w1124, "error in (no error)"=w1125) -> ("error out"=w1121:errorcluster)  [unwired: 13 in]
            n83 = call "GEA2 Write ERD.vi"("GEA2 Reference In"=w1115, "Read Timeout (ms)"=u32 2000, "GEA Inputs"=w1117, "Write ERD List"=w1120, "Error In"=w1121, "Verify ERD Response?"=FALSE) -> ("GEA2 Reference Out"=w1114:refnum<k24>, "Error Out"=w1113:errorcluster)  [unwired: 7 in, 1 out]
          }
          event "Door Lock.Lock Door", "Door Lock.Unlock Door": Value Change {
            n84 = event-data() -> ("CtlRef"=w1129:refnum<vi>)  [unwired: 1 in, 5 out]
            n85 = property class="Bool"(reference=w1129, error in=w1132) -> (reference out=w1135:refnum<vi>, error out=w1136:errorcluster, "Label.Text"=w1137:string)
            n86 = Close Reference(reference=w1135, error in (no error)=w1136) -> (error out=w1134:errorcluster)
            n87 = case shown="\"Lock Door\"" w1137 {
              tunnel: [w1142 w1168] -> w1128
              tunnel: w1131 -> [w1143 w1167]
              tunnel: w1134 -> [w1144 w1159]
              tunnel: w1130 -> [w1141 w1158]
              tunnel: [w1140 w1157] -> _
              tunnel: T28 {"ERD Number"=61441, "Data Type"=enum."string", "Data"=""} ("ERD Read Data In") -> [w1138 w1155]
              frame "Unlock Door", Default {
                n88 = Concatenate Strings("00" ("string")) -> (w1154:string)
                n89 = Bundle By Name(cluster=w1138, "Data"=w1154) -> (w1153:T28)
                n90 = Build Array(w1153) -> (w1146:T28[])
                n91 = call "Convert Write ERD List to Message.vi"("GEA Inputs"=w1141, "Write ERD List"=w1146, "Error In"=w1144) -> ("GEA Message"=w1148:T5, "Error Out"=w1149:errorcluster)  [unwired: 11 in]
                n92 = call "GEA2MessageFormatter.vi"("Prefix(Send/Recv)"="SEND", "GEA2 Data In"=w1148, "Error In"=w1149) -> ("Output String"=w1150:string, "Error Out"=w1151:errorcluster)  [unwired: 11 in]
                n93 = call "GExplorer_Queue_GEA2.vi"("Output String"=w1150, "error in (no error)"=w1151) -> ("error out"=w1147:errorcluster)  [unwired: 13 in]
                n94 = call "GEA2 Write ERD.vi"("GEA2 Reference In"=w1143, "GEA Inputs"=w1141, "Write ERD List"=w1146, "Error In"=w1147, "Verify ERD Response?"=TRUE) -> ("GEA2 Reference Out"=w1140:refnum<k24>, "Error Out"=w1142:errorcluster)  [unwired: 8 in, 1 out]
              }
              frame "Lock Door" {
                n95 = Concatenate Strings("01" ("string")) -> (w1171:string)
                n96 = Bundle By Name(cluster=w1155, "Data"=w1171) -> (w1170:T28)
                n97 = Build Array(w1170) -> (w1161:T28[])
                n98 = call "Convert Write ERD List to Message.vi"("GEA Inputs"=w1158, "Write ERD List"=w1161, "Error In"=w1159) -> ("GEA Message"=w1163:T5, "Error Out"=w1164:errorcluster)  [unwired: 11 in]
                n99 = call "GEA2MessageFormatter.vi"("Prefix(Send/Recv)"="SEND", "GEA2 Data In"=w1163, "Error In"=w1164) -> ("Output String"=w1165:string, "Error Out"=w1166:errorcluster)  [unwired: 11 in]
                n100 = call "GExplorer_Queue_GEA2.vi"("Output String"=w1165, "error in (no error)"=w1166) -> ("error out"=w1162:errorcluster)  [unwired: 13 in]
                n101 = call "GEA2 Write ERD.vi"("GEA2 Reference In"=w1167, "GEA Inputs"=w1158, "Write ERD List"=w1161, "Error In"=w1162, "Verify ERD Response?"=TRUE) -> ("GEA2 Reference Out"=w1157:refnum<k24>, "Error Out"=w1168:errorcluster)  [unwired: 8 in, 1 out]
              }
            }
          }
          event "Drain Pump.ON", "Drain Pump.OFF": Value Change {
            n102 = event-data() -> ("CtlRef"=w1173:refnum<vi>)  [unwired: 1 in, 5 out]
            n103 = property class="Bool"(reference=w1173, error in=w1176) -> (reference out=w1179:refnum<vi>, error out=w1180:errorcluster, "Label.Text"=w1181:string)
            n104 = Close Reference(reference=w1179, error in (no error)=w1180) -> (error out=w1178:errorcluster)
            n105 = case shown="\"ON\"" w1181 {
              tunnel: [w1186 w1212] -> w1172
              tunnel: w1175 -> [w1187 w1211]
              tunnel: w1178 -> [w1188 w1203]
              tunnel: w1174 -> [w1185 w1202]
              tunnel: [w1184 w1201] -> _
              tunnel: T28 {"ERD Number"=61451, "Data Type"=enum."string", "Data"=""} ("ERD Read Data In") -> [w1182 w1199]
              frame "OFF", Default {
                n106 = Concatenate Strings("00" ("string")) -> (w1198:string)
                n107 = Bundle By Name(cluster=w1182, "Data"=w1198) -> (w1197:T28)
                n108 = Build Array(w1197) -> (w1190:T28[])
                n109 = call "Convert Write ERD List to Message.vi"("GEA Inputs"=w1185, "Write ERD List"=w1190, "Error In"=w1188) -> ("GEA Message"=w1192:T5, "Error Out"=w1193:errorcluster)  [unwired: 11 in]
                n110 = call "GEA2MessageFormatter.vi"("Prefix(Send/Recv)"="SEND", "GEA2 Data In"=w1192, "Error In"=w1193) -> ("Output String"=w1194:string, "Error Out"=w1195:errorcluster)  [unwired: 11 in]
                n111 = call "GExplorer_Queue_GEA2.vi"("Output String"=w1194, "error in (no error)"=w1195) -> ("error out"=w1191:errorcluster)  [unwired: 13 in]
                n112 = call "GEA2 Write ERD.vi"("GEA2 Reference In"=w1187, "GEA Inputs"=w1185, "Write ERD List"=w1190, "Error In"=w1191, "Verify ERD Response?"=TRUE) -> ("GEA2 Reference Out"=w1184:refnum<k24>, "Error Out"=w1186:errorcluster)  [unwired: 8 in, 1 out]
              }
              frame "ON" {
                n113 = Concatenate Strings("08" ("string")) -> (w1215:string)
                n114 = Bundle By Name(cluster=w1199, "Data"=w1215) -> (w1214:T28)
                n115 = Build Array(w1214) -> (w1205:T28[])
                n116 = call "Convert Write ERD List to Message.vi"("GEA Inputs"=w1202, "Write ERD List"=w1205, "Error In"=w1203) -> ("GEA Message"=w1207:T5, "Error Out"=w1208:errorcluster)  [unwired: 11 in]
                n117 = call "GEA2MessageFormatter.vi"("Prefix(Send/Recv)"="SEND", "GEA2 Data In"=w1207, "Error In"=w1208) -> ("Output String"=w1209:string, "Error Out"=w1210:errorcluster)  [unwired: 11 in]
                n118 = call "GExplorer_Queue_GEA2.vi"("Output String"=w1209, "error in (no error)"=w1210) -> ("error out"=w1206:errorcluster)  [unwired: 13 in]
                n119 = call "GEA2 Write ERD.vi"("GEA2 Reference In"=w1211, "GEA Inputs"=w1202, "Write ERD List"=w1205, "Error In"=w1206, "Verify ERD Response?"=TRUE) -> ("GEA2 Reference Out"=w1201:refnum<k24>, "Error Out"=w1212:errorcluster)  [unwired: 8 in, 1 out]
              }
            }
          }
          event "Heater.ON", "Heater.OFF": Value Change {
            n120 = event-data() -> ("CtlRef"=w1217:refnum<vi>)  [unwired: 1 in, 5 out]
            n121 = property class="Bool"(reference=w1217, error in=w1220) -> (reference out=w1223:refnum<vi>, error out=w1224:errorcluster, "Label.Text"=w1225:string)
            n122 = Close Reference(reference=w1223, error in (no error)=w1224) -> (error out=w1222:errorcluster)
            n123 = case shown="\"ON\"" w1225 {
              tunnel: [w1230 w1256] -> w1216
              tunnel: w1219 -> [w1231 w1255]
              tunnel: w1222 -> [w1232 w1247]
              tunnel: w1218 -> [w1229 w1246]
              tunnel: [w1228 w1245] -> _
              tunnel: T28 {"ERD Number"=61450, "Data Type"=enum."string", "Data"=""} ("ERD Read Data In") -> [w1226 w1243]
              frame "OFF", Default {
                n124 = Concatenate Strings("00" ("string")) -> (w1242:string)
                n125 = Bundle By Name(cluster=w1226, "Data"=w1242) -> (w1241:T28)
                n126 = Build Array(w1241) -> (w1234:T28[])
                n127 = call "Convert Write ERD List to Message.vi"("GEA Inputs"=w1229, "Write ERD List"=w1234, "Error In"=w1232) -> ("GEA Message"=w1236:T5, "Error Out"=w1237:errorcluster)  [unwired: 11 in]
                n128 = call "GEA2MessageFormatter.vi"("Prefix(Send/Recv)"="SEND", "GEA2 Data In"=w1236, "Error In"=w1237) -> ("Output String"=w1238:string, "Error Out"=w1239:errorcluster)  [unwired: 11 in]
                n129 = call "GExplorer_Queue_GEA2.vi"("Output String"=w1238, "error in (no error)"=w1239) -> ("error out"=w1235:errorcluster)  [unwired: 13 in]
                n130 = call "GEA2 Write ERD.vi"("GEA2 Reference In"=w1231, "GEA Inputs"=w1229, "Write ERD List"=w1234, "Error In"=w1235, "Verify ERD Response?"=TRUE) -> ("GEA2 Reference Out"=w1228:refnum<k24>, "Error Out"=w1230:errorcluster)  [unwired: 8 in, 1 out]
              }
              frame "ON" {
                n131 = Concatenate Strings("02" ("string")) -> (w1259:string)
                n132 = Bundle By Name(cluster=w1243, "Data"=w1259) -> (w1258:T28)
                n133 = Build Array(w1258) -> (w1249:T28[])
                n134 = call "Convert Write ERD List to Message.vi"("GEA Inputs"=w1246, "Write ERD List"=w1249, "Error In"=w1247) -> ("GEA Message"=w1251:T5, "Error Out"=w1252:errorcluster)  [unwired: 11 in]
                n135 = call "GEA2MessageFormatter.vi"("Prefix(Send/Recv)"="SEND", "GEA2 Data In"=w1251, "Error In"=w1252) -> ("Output String"=w1253:string, "Error Out"=w1254:errorcluster)  [unwired: 11 in]
                n136 = call "GExplorer_Queue_GEA2.vi"("Output String"=w1253, "error in (no error)"=w1254) -> ("error out"=w1250:errorcluster)  [unwired: 13 in]
                n137 = call "GEA2 Write ERD.vi"("GEA2 Reference In"=w1255, "GEA Inputs"=w1246, "Write ERD List"=w1249, "Error In"=w1250, "Verify ERD Response?"=TRUE) -> ("GEA2 Reference Out"=w1245:refnum<k24>, "Error Out"=w1256:errorcluster)  [unwired: 8 in, 1 out]
              }
            }
          }
          event Value Change {
            n138 = event-data() -> ("CtlRef"=w1263:refnum<vi>)  [unwired: 1 in, 5 out]
            n139 = property class="Bool"(reference=w1263, error in=w1266) -> (reference out=w1269:refnum<vi>, error out=w1270:errorcluster, "Label.Text"=w1271:string)
            n140 = Close Reference(reference=w1269, error in (no error)=w1270) -> (error out=w1268:errorcluster)
            n141 = case shown="\"Valves ON\"" w1271 {
              tunnel: [w1285 w1327] -> w1262
              tunnel: w1265 -> [w1286 w1326]
              tunnel: w1268 -> [w1287 w1318]
              tunnel: w1264 -> [w1284 w1317]
              tunnel: [w1283 w1316] -> _
              tunnel: T28 {"ERD Number"=61451, "Data Type"=enum."string", "Data"=""} ("ERD Read Data In") -> [w1281 w1314]
              tunnel: T28 {"ERD Number"=61450, "Data Type"=enum."string", "Data"=""} ("ERD Read Data In") -> [w1278 w1300]
              tunnel: "Valve Control" -> [_ w1313]
              frame "Valves OFF", Default {
                n142 = Concatenate Strings("00" ("string")) -> (w1279:string)
                n143 = Concatenate Strings("00" ("string")) -> (w1297:string)
                n144 = Bundle By Name(cluster=w1278, "Data"=w1279) -> (w1277:T28)
                n145 = Bundle By Name(cluster=w1281, "Data"=w1297) -> (w1296:T28)
                n146 = Build Array(w1296, w1277) -> (w1289:T28[])
                n147 = call "Convert Write ERD List to Message.vi"("GEA Inputs"=w1284, "Write ERD List"=w1289, "Error In"=w1287) -> ("GEA Message"=w1291:T5, "Error Out"=w1292:errorcluster)  [unwired: 11 in]
                n148 = property on="Bleach Valve" class="Bool (strict)"("Value"=FALSE) -> ()  [unwired: 2 in, 2 out]
                n149 = property on="PreWash Valve" class="Bool (strict)"("Value"=FALSE) -> ()  [unwired: 2 in, 2 out]
                n150 = call "GEA2MessageFormatter.vi"("Prefix(Send/Recv)"="SEND", "GEA2 Data In"=w1291, "Error In"=w1292) -> ("Output String"=w1293:string, "Error Out"=w1294:errorcluster)  [unwired: 11 in]
                n151 = property on="Hot Valve" class="Bool (strict)"("Value"=FALSE) -> ()  [unwired: 2 in, 2 out]
                n152 = property on="MainWash Valve" class="Bool (strict)"("Value"=FALSE) -> ()  [unwired: 2 in, 2 out]
                n153 = call "GExplorer_Queue_GEA2.vi"("Output String"=w1293, "error in (no error)"=w1294) -> ("error out"=w1290:errorcluster)  [unwired: 13 in]
                n154 = call "GEA2 Write ERD.vi"("GEA2 Reference In"=w1286, "GEA Inputs"=w1284, "Write ERD List"=w1289, "Error In"=w1290, "Verify ERD Response?"=TRUE) -> ("GEA2 Reference Out"=w1283:refnum<k24>, "Error Out"=w1285:errorcluster)  [unwired: 8 in, 1 out]
                n155 = property on="Fabric Softener" class="Bool (strict)"("Value"=FALSE) -> ()  [unwired: 2 in, 2 out]
              }
              frame "Valves ON" {
                n156 = Unbundle By Name(w1313) -> ("Fabric Softener"=w1298:bool, "PreWash Valve"=w1299:bool, "MainWash Valve"=w1312:bool, "Bleach Valve"=w1311:bool, "Hot Valve"=w1305:bool)
                n157 = case shown="False" w1298 {
                  tunnel: w1312 -> [w1333 w1336]
                  tunnel: w1311 -> [w1332 _]
                  tunnel: [w1331 w1337] -> w1310
                  tunnel: w1299 -> [w1330 _]
                  frame False {
                    n158 = Build Array(w1330, w1333, w1332) -> (w1331:bool[])
                  }
                  frame True {
                    n159 = Build Array(TRUE ("element"), w1336, TRUE ("element")) -> (w1337:bool[])
                  }
                }
                n160 = Select(t="20", s=w1305, f="00") -> (s? t:f=w1302:string)
                n161 = Boolean Array To Number(Boolean array=w1310) -> (number=w1309:u32)
                n162 = Number To Hexadecimal String(1:i16 2 ("width (-)"), 2:w1309) -> (0:w1307:string)
                n163 = Concatenate Strings(w1307) -> (w1329:string)
                n164 = Concatenate Strings(w1302) -> (w1306:string)
                n165 = Bundle By Name(cluster=w1314, "Data"=w1329) -> (w1328:T28)
                n166 = Bundle By Name(cluster=w1300, "Data"=w1306) -> (w1301:T28)
                n167 = Build Array(w1328, w1301) -> (w1320:T28[])
                n168 = call "Convert Write ERD List to Message.vi"("GEA Inputs"=w1317, "Write ERD List"=w1320, "Error In"=w1318) -> ("GEA Message"=w1322:T5, "Error Out"=w1323:errorcluster)  [unwired: 11 in]
                n169 = call "GEA2MessageFormatter.vi"("Prefix(Send/Recv)"="SEND", "GEA2 Data In"=w1322, "Error In"=w1323) -> ("Output String"=w1324:string, "Error Out"=w1325:errorcluster)  [unwired: 11 in]
                n170 = call "GExplorer_Queue_GEA2.vi"("Output String"=w1324, "error in (no error)"=w1325) -> ("error out"=w1321:errorcluster)  [unwired: 13 in]
                n171 = call "GEA2 Write ERD.vi"("GEA2 Reference In"=w1326, "GEA Inputs"=w1317, "Write ERD List"=w1320, "Error In"=w1321, "Verify ERD Response?"=TRUE) -> ("GEA2 Reference Out"=w1316:refnum<k24>, "Error Out"=w1327:errorcluster)  [unwired: 8 in, 1 out]
              }
            }
          }
          event Value Change {
            w1350 = TRUE ("Value")
            n172 = event-data() -> ()  [unwired: 1 in, 6 out]
            n173 = property on="Program Ind" class="Bool (strict)"(error in=w1351, "Value"=w1350, "Blinking"=w1350) -> (error out=w1349:errorcluster)  [unwired: 1 in, 1 out]
            n174 = Enqueue Element(queue=w1338, element=T25 {"Data"=variant, "State"=enum."Pause"}, error in (no error)=w1349) -> (error out=w1345:errorcluster)  [unwired: 1 in, 2 out]
            n175 = Unbundle By Name("Programming") -> ("File Path"=w1340:path)
            n176 = Not Equal?(x=w1340, y=path "") -> (x != y?=w1344:bool)
            n177 = case shown="True" w1344 {
              tunnel: w1345 -> [w1353 w1363]
              tunnel: w1343 -> [_ w1372]
              tunnel: w1342 -> [w1352 w1369]
              tunnel: [w1352 w1368] -> w1341
              tunnel: w1340 -> [_ w1367]
              tunnel: [w1353 w1356] -> w1339
              tunnel: w1338 -> [_ w1355]
              frame False {
              }
              frame True {
                w1361 = FALSE ("Value")
                w1365 = T4 9 items=["ImageRejected", "BoardNotFound", "UnableToGetGeaConfiguration", "WriteToFlashNotAllowed", "ImageDownloadedSuccessfully", "ImagePresent", "WriteToFlashFailed", "EraseFailed", "CrcFailed", ""] ("Value")
                n178 = Unbundle By Name(w1372) -> ("Source"=w1371:u8, "Destination"=w1370:u8)
                n179 = property on="Result" class="Ring (strict)"(error in=w1363, "Value"=w1365) -> (error out=w1366:errorcluster)  [unwired: 1 in, 1 out]
                n180 = call "GEA2 Flash APL.vi"("GEA2 Reference In"=w1369, "Force Update?"=TRUE, "Source Address"=w1371, "Destination Address"=w1370, "File Path"=w1367, "Error In"=w1366, "Broadcast"=TRUE, "Reset?"=FALSE ("Reset Board?")) -> ("GEA2 Reference Out"=w1368:refnum<k24>, "Result"=w1360:i32, "Error Out"=w1359:errorcluster)  [unwired: 3 in, 2 out]
                n181 = property on="Board Index" class="DigNum (strict)"(error in=w1363, "DisabledEnum"=T29."Disabled and Grayed Out" ("Disabled")) -> ()  [unwired: 1 in, 2 out]
                n182 = property on="Result" class="Ring (strict)"(error in=w1359, "Value"=w1360) -> (error out=w1358:errorcluster)  [unwired: 1 in, 1 out]
                n183 = property on="Program Ind" class="Bool (strict)"(error in=w1358, "Value"=w1361, "Blinking"=w1361) -> (error out=w1357:errorcluster)  [unwired: 1 in, 1 out]
                n184 = property on="Board Index" class="DigNum (strict)"(error in=w1358, "DisabledEnum"=T29."Enabled" ("Disabled")) -> ()  [unwired: 1 in, 2 out]
                n185 = Enqueue Element(queue=w1355, element=T25 {"Data"=variant, "State"=enum."Init"}, error in (no error)=w1357) -> (error out=w1356:errorcluster)  [unwired: 1 in, 2 out]
              }
            }
          }
          event Value Change {
            n186 = event-data() -> ()  [unwired: 1 in, 6 out]
            n187 = Unbundle By Name(w1391) -> ("Source"=w1377:u8, "Destination"=w1389:u8)
            n188 = Bundle By Name(cluster=T5 {"Source"=228, "Destination"=52, "Command"=221, "Message"="F401"} ("Input Data"), "Source"=w1377, "Destination"=w1389, "Command"=u8 221, "Message"="07") -> (w1390:T5)
            n189 = call "GEA2 Send Message.vi"("GEA2 Reference In"=w1395, "Input Data"=w1390, "Error In"=w1396) -> ("GEA2 Reference Out"=w1379:refnum<k24>, "Error Out"=w1400:errorcluster)  [unwired: 11 in]
            n190 = call "GEA2MessageFormatter.vi"("Prefix(Send/Recv)"="SEND", "GEA2 Data In"=w1390, "Error In"=w1400) -> ("Output String"=w1398:string, "Error Out"=w1397:errorcluster)  [unwired: 11 in]
            n191 = call "GExplorer_Queue_GEA2.vi"("Output String"=w1398, "error in (no error)"=w1397) -> ("error out"=w1380:errorcluster)  [unwired: 13 in]
            n192 = Bundle By Name(cluster=T5 {"Source"=228, "Destination"=52, "Command"=221, "Message"="F401"} ("Input Data"), "Source"=w1377, "Destination"=u8 255, "Command"=u8 221, "Message"="07") -> (w1381:T5)
            n193 = call "GEA2 Send Message.vi"("GEA2 Reference In"=w1379, "Input Data"=w1381, "Error In"=w1380) -> ("Error Out"=w1388:errorcluster)  [unwired: 11 in, 1 out]
            n194 = call "GEA2MessageFormatter.vi"("Prefix(Send/Recv)"="SEND", "GEA2 Data In"=w1381, "Error In"=w1388) -> ("Output String"=w1386:string, "Error Out"=w1385:errorcluster)  [unwired: 11 in]
            n195 = call "GExplorer_Queue_GEA2.vi"("Output String"=w1386, "error in (no error)"=w1385) -> ("error out"=w1378:errorcluster)  [unwired: 13 in]
          }
          event Value Change {
            n196 = event-data() -> ()  [unwired: 1 in, 6 out]
            n197 = Unbundle By Name(w1422) -> ("Source"=w1403:u8, "Destination"=w1414:u8)
            n198 = Bundle By Name(cluster=T5 {"Source"=228, "Destination"=52, "Command"=221, "Message"="F401"} ("Input Data"), "Source"=w1403, "Destination"=w1414, "Command"=u8 221, "Message"="F4 01") -> (w1420:T5)
            n199 = call "GEA2 Send Message.vi"("GEA2 Reference In"=w1424, "Input Data"=w1420, "Error In"=w1425) -> ("GEA2 Reference Out"=w1401:refnum<k24>, "Error Out"=w1430:errorcluster)  [unwired: 11 in]
            n200 = call "GEA2MessageFormatter.vi"("Prefix(Send/Recv)"="SEND", "GEA2 Data In"=w1420, "Error In"=w1430) -> ("Output String"=w1428:string, "Error Out"=w1427:errorcluster)  [unwired: 11 in]
            n201 = call "GExplorer_Queue_GEA2.vi"("Output String"=w1428, "error in (no error)"=w1427) -> ("error out"=w1405:errorcluster)  [unwired: 13 in]
            n202 = Bundle By Name(cluster=T5 {"Source"=228, "Destination"=52, "Command"=221, "Message"="F401"} ("Input Data"), "Source"=w1403, "Destination"=u8 255, "Command"=u8 221, "Message"="F4 01") -> (w1412:T5)
            n203 = call "GEA2 Send Message.vi"("GEA2 Reference In"=w1401, "Input Data"=w1412, "Error In"=w1405) -> ("Error Out"=w1406:errorcluster)  [unwired: 11 in, 1 out]
            n204 = call "GEA2MessageFormatter.vi"("Prefix(Send/Recv)"="SEND", "GEA2 Data In"=w1412, "Error In"=w1406) -> ("Output String"=w1408:string, "Error Out"=w1409:errorcluster)  [unwired: 11 in]
            n205 = call "GExplorer_Queue_GEA2.vi"("Output String"=w1408, "error in (no error)"=w1409) -> ("error out"=w1404:errorcluster)  [unwired: 13 in]
            n206 = call "Time Delay2"("error in (no error)"=w1404, "Delay Time (s)"=2.0) -> ("error out"=w1418:errorcluster)  [unwired: 9 in]
            n207 = Enqueue Element(queue=w1415, element=T25 {"Data"=variant, "State"=enum."Init"} ("Data"), error in (no error)=w1418) -> (error out=w1417:errorcluster)  [unwired: 1 in, 2 out]
          }
          event "Drum Light.ON", "Drum Light.OFF": Value Change {
            n208 = event-data() -> ("CtlRef"=w1432:refnum<vi>)  [unwired: 1 in, 5 out]
            n209 = property class="Bool"(reference=w1432, error in=w1435) -> (reference out=w1438:refnum<vi>, error out=w1439:errorcluster, "Label.Text"=w1440:string)
            n210 = Close Reference(reference=w1438, error in (no error)=w1439) -> (error out=w1437:errorcluster)
            n211 = case shown="\"OFF\", Default" w1440 {
              tunnel: [w1445 w1471] -> w1431
              tunnel: w1434 -> [w1446 w1470]
              tunnel: w1437 -> [w1447 w1462]
              tunnel: w1433 -> [w1444 w1461]
              tunnel: [w1443 w1460] -> _
              tunnel: T28 {"ERD Number"=61448, "Data Type"=enum."string", "Data"=""} ("ERD Read Data In") -> [w1441 w1458]
              frame "OFF", Default {
                n212 = Concatenate Strings("00" ("string")) -> (w1457:string)
                n213 = Bundle By Name(cluster=w1441, "Data"=w1457) -> (w1456:T28)
                n214 = Build Array(w1456) -> (w1449:T28[])
                n215 = call "Convert Write ERD List to Message.vi"("GEA Inputs"=w1444, "Write ERD List"=w1449, "Error In"=w1447) -> ("GEA Message"=w1451:T5, "Error Out"=w1452:errorcluster)  [unwired: 11 in]
                n216 = call "GEA2MessageFormatter.vi"("Prefix(Send/Recv)"="SEND", "GEA2 Data In"=w1451, "Error In"=w1452) -> ("Output String"=w1453:string, "Error Out"=w1454:errorcluster)  [unwired: 11 in]
                n217 = call "GExplorer_Queue_GEA2.vi"("Output String"=w1453, "error in (no error)"=w1454) -> ("error out"=w1450:errorcluster)  [unwired: 13 in]
                n218 = call "GEA2 Write ERD.vi"("GEA2 Reference In"=w1446, "GEA Inputs"=w1444, "Write ERD List"=w1449, "Error In"=w1450, "Verify ERD Response?"=TRUE) -> ("GEA2 Reference Out"=w1443:refnum<k24>, "Error Out"=w1445:errorcluster)  [unwired: 8 in, 1 out]
              }
              frame "ON" {
                n219 = Concatenate Strings("01" ("string")) -> (w1474:string)
                n220 = Bundle By Name(cluster=w1458, "Data"=w1474) -> (w1473:T28)
                n221 = Build Array(w1473) -> (w1464:T28[])
                n222 = call "Convert Write ERD List to Message.vi"("GEA Inputs"=w1461, "Write ERD List"=w1464, "Error In"=w1462) -> ("GEA Message"=w1466:T5, "Error Out"=w1467:errorcluster)  [unwired: 11 in]
                n223 = call "GEA2MessageFormatter.vi"("Prefix(Send/Recv)"="SEND", "GEA2 Data In"=w1466, "Error In"=w1467) -> ("Output String"=w1468:string, "Error Out"=w1469:errorcluster)  [unwired: 11 in]
                n224 = call "GExplorer_Queue_GEA2.vi"("Output String"=w1468, "error in (no error)"=w1469) -> ("error out"=w1465:errorcluster)  [unwired: 13 in]
                n225 = call "GEA2 Write ERD.vi"("GEA2 Reference In"=w1470, "GEA Inputs"=w1461, "Write ERD List"=w1464, "Error In"=w1465, "Verify ERD Response?"=TRUE) -> ("GEA2 Reference Out"=w1460:refnum<k24>, "Error Out"=w1471:errorcluster)  [unwired: 8 in, 1 out]
              }
            }
          }
          event "LEDs.ON", "LEDs.OFF": Value Change {
            n226 = event-data() -> ("CtlRef"=w1476:refnum<vi>)  [unwired: 1 in, 5 out]
            n227 = property class="Bool"(reference=w1476, error in=w1479) -> (reference out=w1482:refnum<vi>, error out=w1483:errorcluster, "Label.Text"=w1484:string)
            n228 = Close Reference(reference=w1482, error in (no error)=w1483) -> (error out=w1481:errorcluster)
            n229 = case shown="\"ON\"" w1484 {
              tunnel: [w1489 w1515] -> w1475
              tunnel: w1478 -> [w1490 w1514]
              tunnel: w1481 -> [w1491 w1506]
              tunnel: w1477 -> [w1488 w1505]
              tunnel: [w1487 w1504] -> _
              tunnel: T28 {"ERD Number"=61447, "Data Type"=enum."string", "Data"=""} ("ERD Read Data In") -> [w1485 w1502]
              frame "OFF", Default {
                n230 = Concatenate Strings("00 00 00 00 00 00 00 00 00 00 00" ("string")) -> (w1501:string)
                n231 = Bundle By Name(cluster=w1485, "Data"=w1501) -> (w1500:T28)
                n232 = Build Array(w1500) -> (w1493:T28[])
                n233 = call "Convert Write ERD List to Message.vi"("GEA Inputs"=w1488, "Write ERD List"=w1493, "Error In"=w1491) -> ("GEA Message"=w1495:T5, "Error Out"=w1496:errorcluster)  [unwired: 11 in]
                n234 = call "GEA2MessageFormatter.vi"("Prefix(Send/Recv)"="SEND", "GEA2 Data In"=w1495, "Error In"=w1496) -> ("Output String"=w1497:string, "Error Out"=w1498:errorcluster)  [unwired: 11 in]
                n235 = call "GExplorer_Queue_GEA2.vi"("Output String"=w1497, "error in (no error)"=w1498) -> ("error out"=w1494:errorcluster)  [unwired: 13 in]
                n236 = call "GEA2 Write ERD.vi"("GEA2 Reference In"=w1490, "GEA Inputs"=w1488, "Write ERD List"=w1493, "Error In"=w1494, "Verify ERD Response?"=TRUE) -> ("GEA2 Reference Out"=w1487:refnum<k24>, "Error Out"=w1489:errorcluster)  [unwired: 8 in, 1 out]
              }
              frame "ON" {
                n237 = Concatenate Strings("FF FF FF FF FF FF FF FF FF FF FF" ("string")) -> (w1518:string)
                n238 = Bundle By Name(cluster=w1502, "Data"=w1518) -> (w1517:T28)
                n239 = Build Array(w1517) -> (w1508:T28[])
                n240 = call "Convert Write ERD List to Message.vi"("GEA Inputs"=w1505, "Write ERD List"=w1508, "Error In"=w1506) -> ("GEA Message"=w1510:T5, "Error Out"=w1511:errorcluster)  [unwired: 11 in]
                n241 = call "GEA2MessageFormatter.vi"("Prefix(Send/Recv)"="SEND", "GEA2 Data In"=w1510, "Error In"=w1511) -> ("Output String"=w1512:string, "Error Out"=w1513:errorcluster)  [unwired: 11 in]
                n242 = call "GExplorer_Queue_GEA2.vi"("Output String"=w1512, "error in (no error)"=w1513) -> ("error out"=w1509:errorcluster)  [unwired: 13 in]
                n243 = call "GEA2 Write ERD.vi"("GEA2 Reference In"=w1514, "GEA Inputs"=w1505, "Write ERD List"=w1508, "Error In"=w1509, "Verify ERD Response?"=TRUE) -> ("GEA2 Reference Out"=w1504:refnum<k24>, "Error Out"=w1515:errorcluster)  [unwired: 8 in, 1 out]
              }
            }
          }
          event "Buzzer.Test": Value Change {
            n244 = event-data() -> ("CtlRef"=w1520:refnum<vi>)  [unwired: 1 in, 5 out]
            n245 = property class="Bool"(reference=w1520, error in=w1523) -> (reference out=w1526:refnum<vi>, error out=w1527:errorcluster, "Label.Text"=w1528:string)
            n246 = Close Reference(reference=w1526, error in (no error)=w1527) -> (error out=w1525:errorcluster)
            n247 = case shown="\"Test\", Default" w1528 {
              tunnel: [w1533] -> w1519
              tunnel: w1522 -> [w1534]
              tunnel: w1525 -> [w1535]
              tunnel: w1521 -> [w1532]
              tunnel: [w1531] -> _
              tunnel: T28 {"ERD Number"=61449, "Data Type"=enum."string", "Data"=""} ("ERD Read Data In") -> [w1529]
              frame "Test", Default {
                n248 = Concatenate Strings("FF" ("string")) -> (w1545:string)
                n249 = Bundle By Name(cluster=w1529, "Data"=w1545) -> (w1544:T28)
                n250 = Build Array(w1544) -> (w1537:T28[])
                n251 = call "Convert Write ERD List to Message.vi"("GEA Inputs"=w1532, "Write ERD List"=w1537, "Error In"=w1535) -> ("GEA Message"=w1539:T5, "Error Out"=w1540:errorcluster)  [unwired: 11 in]
                n252 = call "GEA2MessageFormatter.vi"("Prefix(Send/Recv)"="SEND", "GEA2 Data In"=w1539, "Error In"=w1540) -> ("Output String"=w1541:string, "Error Out"=w1542:errorcluster)  [unwired: 11 in]
                n253 = call "GExplorer_Queue_GEA2.vi"("Output String"=w1541, "error in (no error)"=w1542) -> ("error out"=w1538:errorcluster)  [unwired: 13 in]
                n254 = call "GEA2 Write ERD.vi"("GEA2 Reference In"=w1534, "GEA Inputs"=w1532, "Write ERD List"=w1537, "Error In"=w1538, "Verify ERD Response?"=TRUE) -> ("GEA2 Reference Out"=w1531:refnum<k24>, "Error Out"=w1533:errorcluster)  [unwired: 8 in, 1 out]
              }
            }
          }
          event "Test Mode.Exit", "Test Mode.Enter": Value Change {
            n255 = event-data() -> ("CtlRef"=w1547:refnum<vi>)  [unwired: 1 in, 5 out]
            n256 = property class="Bool"(reference=w1547, error in=w1550) -> (reference out=w1553:refnum<vi>, error out=w1554:errorcluster, "Label.Text"=w1555:string)
            n257 = Close Reference(reference=w1553, error in (no error)=w1554) -> (error out=w1552:errorcluster)
            n258 = case shown="\"Exit\"" w1555 {
              tunnel: [w1560 w1586] -> w1546
              tunnel: w1549 -> [w1561 w1585]
              tunnel: w1552 -> [w1562 w1577]
              tunnel: w1548 -> [w1559 w1576]
              tunnel: [w1558 w1575] -> _
              tunnel: T28 {"ERD Number"=61440, "Data Type"=enum."string", "Data"=""} ("ERD Read Data In") -> [w1556 w1573]
              frame "Enter", Default {
                n259 = Concatenate Strings("01" ("string")) -> (w1572:string)
                n260 = Bundle By Name(cluster=w1556, "Data"=w1572) -> (w1571:T28)
                n261 = Build Array(w1571) -> (w1564:T28[])
                n262 = call "Convert Write ERD List to Message.vi"("GEA Inputs"=w1559, "Write ERD List"=w1564, "Error In"=w1562) -> ("GEA Message"=w1566:T5, "Error Out"=w1567:errorcluster)  [unwired: 11 in]
                n263 = call "GEA2MessageFormatter.vi"("Prefix(Send/Recv)"="SEND", "GEA2 Data In"=w1566, "Error In"=w1567) -> ("Output String"=w1568:string, "Error Out"=w1569:errorcluster)  [unwired: 11 in]
                n264 = call "GExplorer_Queue_GEA2.vi"("Output String"=w1568, "error in (no error)"=w1569) -> ("error out"=w1565:errorcluster)  [unwired: 13 in]
                n265 = call "GEA2 Write ERD.vi"("GEA2 Reference In"=w1561, "GEA Inputs"=w1559, "Write ERD List"=w1564, "Error In"=w1565, "Verify ERD Response?"=TRUE) -> ("GEA2 Reference Out"=w1558:refnum<k24>, "Error Out"=w1560:errorcluster)  [unwired: 8 in, 1 out]
              }
              frame "Exit" {
                n266 = Concatenate Strings("00" ("string")) -> (w1589:string)
                n267 = Bundle By Name(cluster=w1573, "Data"=w1589) -> (w1588:T28)
                n268 = Build Array(w1588) -> (w1579:T28[])
                n269 = call "Convert Write ERD List to Message.vi"("GEA Inputs"=w1576, "Write ERD List"=w1579, "Error In"=w1577) -> ("GEA Message"=w1581:T5, "Error Out"=w1582:errorcluster)  [unwired: 11 in]
                n270 = call "GEA2MessageFormatter.vi"("Prefix(Send/Recv)"="SEND", "GEA2 Data In"=w1581, "Error In"=w1582) -> ("Output String"=w1583:string, "Error Out"=w1584:errorcluster)  [unwired: 11 in]
                n271 = call "GExplorer_Queue_GEA2.vi"("Output String"=w1583, "error in (no error)"=w1584) -> ("error out"=w1580:errorcluster)  [unwired: 13 in]
                n272 = call "GEA2 Write ERD.vi"("GEA2 Reference In"=w1585, "GEA Inputs"=w1576, "Write ERD List"=w1579, "Error In"=w1580, "Verify ERD Response?"=TRUE) -> ("GEA2 Reference Out"=w1575:refnum<k24>, "Error Out"=w1586:errorcluster)  [unwired: 8 in, 1 out]
              }
            }
          }
          event Value Change {
            n273 = event-data() -> ("CtlRef"=w1592:refnum<vi>)  [unwired: 1 in, 5 out]
            n274 = property class="Bool"(reference=w1592, error in=w1595) -> (reference out=w1598:refnum<vi>, error out=w1599:errorcluster, "Label.Text"=w1600:string)
            n275 = Close Reference(reference=w1598, error in (no error)=w1599) -> (error out=w1597:errorcluster)
            n276 = case shown="\"Start Motor\", Default" w1600 {
              tunnel: [w1609 w1634] -> w1590
              tunnel: w1594 -> [w1610 w1633]
              tunnel: w1597 -> [w1611 w1625]
              tunnel: w1593 -> [w1608 w1624]
              tunnel: [w1607 w1623] -> _
              tunnel: T28 {"ERD Number"=61444, "Data Type"=enum."string", "Data"=""} ("ERD Read Data In") -> [w1605 w1621]
              tunnel: "Motor Control" -> [w1604 _]
              frame "Start Motor", Default {
                n277 = Unbundle By Name(w1604) -> ("Speed (RPM)"=w1602:i16)
                n278 = Number To Hexadecimal String(1:i16 4 ("width (-)"), 2:w1602) -> (0:w1603:string)
                n279 = Concatenate Strings(w1603) -> (w1620:string)
                n280 = Bundle By Name(cluster=w1605, "Data"=w1620) -> (w1619:T28)
                n281 = Build Array(w1619) -> (w1613:T28[])
                n282 = call "Convert Write ERD List to Message.vi"("GEA Inputs"=w1608, "Write ERD List"=w1613, "Error In"=w1611) -> ("GEA Message"=w1615:T5, "Error Out"=w1616:errorcluster)  [unwired: 11 in]
                n283 = call "GEA2MessageFormatter.vi"("Prefix(Send/Recv)"="SEND", "GEA2 Data In"=w1615, "Error In"=w1616) -> ("Output String"=w1617:string, "Error Out"=w1618:errorcluster)  [unwired: 11 in]
                n284 = call "GExplorer_Queue_GEA2.vi"("Output String"=w1617, "error in (no error)"=w1618) -> ("error out"=w1614:errorcluster)  [unwired: 13 in]
                n285 = call "GEA2 Write ERD.vi"("GEA2 Reference In"=w1610, "GEA Inputs"=w1608, "Write ERD List"=w1613, "Error In"=w1614, "Verify ERD Response?"=TRUE) -> ("GEA2 Reference Out"=w1607:refnum<k24>, "Error Out"=w1609:errorcluster)  [unwired: 8 in, 1 out]
              }
              frame "Stop Motor" {
                n286 = Concatenate Strings("00 00" ("string")) -> (w1637:string)
                n287 = Bundle By Name(cluster=w1621, "Data"=w1637) -> (w1636:T28)
                n288 = Build Array(w1636) -> (w1627:T28[])
                n289 = call "Convert Write ERD List to Message.vi"("GEA Inputs"=w1624, "Write ERD List"=w1627, "Error In"=w1625) -> ("GEA Message"=w1629:T5, "Error Out"=w1630:errorcluster)  [unwired: 11 in]
                n290 = call "GEA2MessageFormatter.vi"("Prefix(Send/Recv)"="SEND", "GEA2 Data In"=w1629, "Error In"=w1630) -> ("Output String"=w1631:string, "Error Out"=w1632:errorcluster)  [unwired: 11 in]
                n291 = call "GExplorer_Queue_GEA2.vi"("Output String"=w1631, "error in (no error)"=w1632) -> ("error out"=w1628:errorcluster)  [unwired: 13 in]
                n292 = call "GEA2 Write ERD.vi"("GEA2 Reference In"=w1633, "GEA Inputs"=w1624, "Write ERD List"=w1627, "Error In"=w1628, "Verify ERD Response?"=TRUE) -> ("GEA2 Reference Out"=w1623:refnum<k24>, "Error Out"=w1634:errorcluster)  [unwired: 8 in, 1 out]
              }
            }
          }
          event "Clear Fault Table Buffer": Value Change {
            n293 = event-data() -> ()  [unwired: 1 in, 6 out]
            n294 = Bundle By Name(cluster=T28 {"ERD Number"=130, "Data Type"=enum."string", "Data"=""} ("ERD Read Data In"), "Data"="FF") -> (w1653:T28)
            n295 = Build Array(w1653) -> (w1647:T28[])
            n296 = call "Convert Write ERD List to Message.vi"("GEA Inputs"=w1644, "Write ERD List"=w1647, "Error In"=w1643) -> ("GEA Message"=w1649:T5, "Error Out"=w1650:errorcluster)  [unwired: 11 in]
            n297 = call "GEA2MessageFormatter.vi"("Prefix(Send/Recv)"="SEND", "GEA2 Data In"=w1649, "Error In"=w1650) -> ("Output String"=w1651:string, "Error Out"=w1652:errorcluster)  [unwired: 11 in]
            n298 = call "GExplorer_Queue_GEA2.vi"("Output String"=w1651, "error in (no error)"=w1652) -> ("error out"=w1648:errorcluster)  [unwired: 13 in]
            n299 = call "GEA2 Write ERD.vi"("GEA2 Reference In"=w1642, "Read Timeout (ms)"=u32 2000, "GEA Inputs"=w1644, "Write ERD List"=w1647, "Error In"=w1648, "Verify ERD Response?"=FALSE) -> ("GEA2 Reference Out"=w1641:refnum<k24>, "Error Out"=w1640:errorcluster)  [unwired: 7 in, 1 out]
          }
          event "Clear Cycle Buffer": Value Change {
            n300 = event-data() -> ()  [unwired: 1 in, 6 out]
            n301 = Build Array(T28 {"ERD Number"=136, "Data Type"=enum."string", "Data"="FF"} ("ERD Read Data In")) -> (w1667:T28[])
            n302 = call "Convert Write ERD List to Message.vi"("GEA Inputs"=w1662, "Write ERD List"=w1667, "Error In"=w1665) -> ("GEA Message"=w1669:T5, "Error Out"=w1670:errorcluster)  [unwired: 11 in]
            n303 = call "GEA2MessageFormatter.vi"("Prefix(Send/Recv)"="SEND", "GEA2 Data In"=w1669, "Error In"=w1670) -> ("Output String"=w1671:string, "Error Out"=w1672:errorcluster)  [unwired: 11 in]
            n304 = call "GExplorer_Queue_GEA2.vi"("Output String"=w1671, "error in (no error)"=w1672) -> ("error out"=w1668:errorcluster)  [unwired: 13 in]
            n305 = call "GEA2 Write ERD.vi"("GEA2 Reference In"=w1664, "GEA Inputs"=w1662, "Write ERD List"=w1667, "Error In"=w1668) -> ("Error Out"=w1661:errorcluster)  [unwired: 9 in, 2 out]
            n306 = call "Time Delay6"("error in (no error)"=w1661) -> ("error out"=w1656:errorcluster)  [unwired: 10 in]
            n307 = property on="Get Cycle History" class="Bool (strict)"(error in=w1656, "Val(Sgnl)"=TRUE ("Get Cycle History")) -> (error out=w1660:errorcluster)  [unwired: 1 in, 1 out]
            n308 = call "Time Delay7"("error in (no error)"=w1660) -> ("error out"=w1655:errorcluster)  [unwired: 10 in]
            n309 = property on="Get Cycle History" class="Bool (strict)"(error in=w1655, "Val(Sgnl)"=FALSE ("Get Cycle History")) -> (error out=w1659:errorcluster)  [unwired: 1 in, 1 out]
          }
          event "Get Cycle History": Value Change {
            w1679 = T8[] [{"ERD Number"=135, "Data Type"=enum."string"}, {"ERD Number"=57344, "Data Type"=enum."string"}, {"ERD Number"=57345, "Data Type"=enum."string"}, {"ERD Number"=57346, "Data Type"=enum."string"}, {"ERD Number"=57347, "Data Type"=enum."string"}, {"ERD Number"=57348, "Data Type"=enum."string"}, {"ERD Number"=57349, "Data Type"=enum."string"}, {"ERD Number"=57350, "Data Type"=enum."string"}, {"ERD Number"=57351, "Data Type"=enum."string"}, {"ERD Number"=57352, "Data Type"=enum."string"}, {"ERD Number"=57353, "Data Type"=enum."string"}] ("Read ERD List")
            n310 = event-data() -> ()  [unwired: 1 in, 6 out]
            n311 = call "Convert Read ERD List to Message.vi"("GEA Inputs"=w1674, "Read ERD List"=w1679, "Error In"=w1681) -> ("GEA Message"=w1685:T5, "Error Out"=w1686:errorcluster)  [unwired: 11 in]
            n312 = call "GEA2MessageFormatter.vi"("Prefix(Send/Recv)"="SEND", "GEA2 Data In"=w1685, "Error In"=w1686) -> ("Output String"=w1684:string, "Error Out"=w1683:errorcluster)  [unwired: 11 in]
            n313 = call "GExplorer_Queue_GEA2.vi"("Output String"=w1684, "error in (no error)"=w1683) -> ("error out"=w1680:errorcluster)  [unwired: 13 in]
            n314 = call "GEA2 Read ERD Multiple Messages.vi"("GEA2 Reference In"=w1675, "Read Timeout (ms)"=u32 500, "GEA Inputs"=w1674, "Read ERD List"=w1679, "Error In"=w1680, "#ERDs per message"=4, "Verify ERD Response?"=TRUE) -> ("ERD Data Out"=w1687:T34[], "Error Out"=w1678:errorcluster)  [unwired: 5 in, 2 out]
            n315 = call "Cycle_Diag_Table_Read_TL24.vi"("ERD Data In"=w1687, "error in (no error)"=w1678) -> ("Cycle Buffer Status"=→"Cycle Buffer Status":T16, "Diag Cycle String Out"=→"Diagnostics Table":string[][], "error out"=w1673:errorcluster)  [unwired: 10 in, 1 out]
          }
          event "Save Cycle History Log": Value Change {
            w1695 = T8[] [{"ERD Number"=135, "Data Type"=enum."string"}, {"ERD Number"=57344, "Data Type"=enum."string"}, {"ERD Number"=57345, "Data Type"=enum."string"}, {"ERD Number"=57346, "Data Type"=enum."string"}, {"ERD Number"=57347, "Data Type"=enum."string"}, {"ERD Number"=57348, "Data Type"=enum."string"}, {"ERD Number"=57349, "Data Type"=enum."string"}, {"ERD Number"=57350, "Data Type"=enum."string"}, {"ERD Number"=57351, "Data Type"=enum."string"}, {"ERD Number"=57352, "Data Type"=enum."string"}, {"ERD Number"=57353, "Data Type"=enum."string"}] ("Read ERD List")
            n316 = event-data() -> ()  [unwired: 1 in, 6 out]
            n317 = call "Convert Read ERD List to Message.vi"("GEA Inputs"=w1698, "Read ERD List"=w1695, "Error In"=w1697) -> ("GEA Message"=w1704:T5, "Error Out"=w1705:errorcluster)  [unwired: 11 in]
            n318 = call "GEA2MessageFormatter.vi"("Prefix(Send/Recv)"="SEND", "GEA2 Data In"=w1704, "Error In"=w1705) -> ("Output String"=w1703:string, "Error Out"=w1702:errorcluster)  [unwired: 11 in]
            n319 = call "GExplorer_Queue_GEA2.vi"("Output String"=w1703, "error in (no error)"=w1702) -> ("error out"=w1700:errorcluster)  [unwired: 13 in]
            n320 = call "GEA2 Read ERD Multiple Messages.vi"("GEA2 Reference In"=w1696, "Read Timeout (ms)"=u32 500, "GEA Inputs"=w1698, "Read ERD List"=w1695, "Error In"=w1700, "#ERDs per message"=4, "Verify ERD Response?"=TRUE) -> ("ERD Data Out"=w1694:T34[], "Error Out"=w1699:errorcluster)  [unwired: 5 in, 2 out]
            n321 = call "Cycle_Diag_Table_Read_TL24.vi"("ERD Data In"=w1694, "error in (no error)"=w1699) -> ("Diag Cycle String Out"=w1693:string[][], "error out"=w1692:errorcluster)  [unwired: 10 in, 2 out]
            n322 = call "Cycle_History_Logging.vi"("error in (no error)"=w1692, "Diag Cycle String Out"=w1693) -> ("error out"=w1691:errorcluster)  [unwired: 9 in]
          }
          event "Data ON": Value Change {
            n323 = event-data() -> ()  [unwired: 1 in, 6 out]
            n324 = case shown="True" "Data ON" {
              tunnel: w1712 -> [w1715 w1719]
              tunnel: [w1714 w1718] -> w1711
              tunnel: w1709 -> [w1713 w1717]
              frame True {
                n325 = Enqueue Element(queue=w1713, element=T25 {"Data"=variant, "State"=enum."Init"} ("Data"), error in (no error)=w1715) -> (error out=w1714:errorcluster)  [unwired: 1 in, 2 out]
              }
              frame False {
                n326 = Enqueue Element(queue=w1717, element=T25 {"Data"=variant, "State"=enum."Pause"} ("Data"), error in (no error)=w1719) -> (error out=w1718:errorcluster)  [unwired: 1 in, 2 out]
              }
            }
          }
          event "Stop": Value Change; User Event; Panel Close {
            n327 = event-data() -> ()  [unwired: 1 in, 3 out]
            n328 = call "Control_ERD_Loop_Brass.vi"("Command (ERD Loop Control)"=ERD_Loop_Control_Command_Brass."Shutdown", "Error In"=w1729) -> ("Error Out"=w1728:errorcluster)  [unwired: 13 in]
            n329 = call "Control_GEA2_Loop_Brass.vi"("Command (ERD Loop Control)"=GEA2_Control_Command_Brass."Shutdown", "Error In"=w1728) -> ("Error Out"=w1730:errorcluster)  [unwired: 13 in]
            n330 = call "Control_DAQ_Loop_Brass.vi"("Command (DAQ Control)"=DAQ_Control_Command_Brass."Shutdown", "Error In"=w1730) -> ("Error Out"=w1733:errorcluster)  [unwired: 13 in]
            n331 = call "Control_Cont_Send_Brass.vi"("Command (ERD Loop Control)"=GEA2_Control_Command_Brass."Shutdown", "Error In"=w1733) -> ("Error Out"=w1723:errorcluster)  [unwired: 13 in]
            n332 = call "Time Delay"("error in (no error)"=w1723, "Delay Time (s)"=2.0) -> ("error out"=w1722:errorcluster)  [unwired: 9 in]
          }
        }
        n333 = call "Error_Control_Brass.vi"("Error In"=w1020) -> ("Error Out"=w1022:errorcluster)  [unwired: 14 in]
      }
      n334 = Unbundle By Name(T25 {"Data"=variant, "State"=enum."Init"} ("Data")) -> ("State"=w73:T26)
      n335 = Build Array(w27, w68, w66, w67, w26, w25, w24) -> (w65:refnum<vi>[])
      n336 = while "DAQ Loop" {
        shift-right: [w495] -> w100
        shift-left: w37 -> [w493]
        shift-right: [w472] -> _
        shift-left: DAQ_States_Brass."Wait for Init" ("States") -> [w490]
        shift-right: [w473] -> _
        shift-left: "Wait for Init" ("Report Text") -> [w488]
        tunnel: w64 -> [w489]
        shift-right: [w471] -> _
        shift-left: _ -> [w428]
        shift-right: [w470] -> _
        shift-left: FALSE -> [w469]
        shift-right: [w459] -> _
        shift-left: w56 -> [w458]
        shift-right: [w457] -> _
        shift-left: w56 -> [w456]
        shift-right: [w455] -> _
        shift-left: w56 -> [w454]
        shift-right: [w453] -> _
        shift-left: w56 -> [w452]
        shift-right: [w451] -> _
        shift-left: w56 -> [w450]
        shift-right: [w449] -> _
        shift-left: w56 -> [w448]
        shift-right: [w447] -> _
        shift-left: w56 -> [w446]
        shift-right: [w433] -> _
        shift-left: 1.0 -> [w429]
        shift-right: [w432] -> _
        shift-left: 1.0 -> [w436]
        shift-right: [w431] -> _
        shift-left: 0.0 -> [w435]
        shift-right: [w427] -> _
        shift-left: w56 -> [w426]
        shift-right: [w425] -> _
        shift-left: FALSE -> [w460]
        stop <- w485 stop-if-true
        # "Automatic Modeshift Feedback"
        # "DAQ Loop"
        n337 = Greater?(x=w436, y=5.0 ("x")) -> (0:w438:bool)
        n338 = Dequeue Element(queue=w489, timeout in ms (-1)=0, error in (no error)=w493) -> (element=w491:T24, timed out?=w492:bool, error out=w484:errorcluster)  [unwired: 1 out]
        n339 = Wait (ms)(milliseconds to wait=u32 250) -> ()  [unwired: 1 out]
        n340 = Select(t="Basket RPM", s=w438, f=w429) -> (s? t:f=w433:dbl)
        n341 = Select(t=w490, s=w492, f=w491) -> (s? t:f=w487:T24)
        n342 = Multiply(x=w433, y=0.40625) -> (x*y=w464:dbl)
        n343 = Less?(x=w433, y=1.0) -> (x < y?=w462:bool)
        n344 = Equal?(x=w429, y=w433) -> (x = y?=w461:bool)
        n345 = case shown="\"Run\"" w487 {
          selector: w487 -> [_ _ _ _ _ _ w974]
          tunnel: [_ _ _ w687 w807 _ _] -> w427
          tunnel: [w527 w551 w583 w688 w805 w912 w977] -> w481
          tunnel: w446 -> [w542 w566 w591 _ w804 w906 w923]
          tunnel: [w542 w566 w591 w692 w803 _ _] -> w447
          tunnel: w448 -> [w541 w565 w592 _ w802 w903 w950]
          tunnel: [w541 w565 w592 w696 w801 _ _] -> w449
          tunnel: [w525 w549 w575 w695 w800 w866 w940] -> w479
          tunnel: [w526 w550 w576 w691 w799 w873 w952] -> w480
          tunnel: [w536 DAQ_States_Brass."Verify Hardware" ("t") w588 DAQ_States_Brass."Run" ("t") w777 DAQ_States_Brass."Wait for Init" ("States") w974] -> w472
          tunnel: [FALSE FALSE FALSE TRUE TRUE FALSE FALSE] -> w471
          tunnel: w454 -> [w540 w564 w595 _ w762 w910 w979]
          tunnel: [w522 w546 w572 w684 w796 w859 w937] -> w476
          tunnel: [w540 w564 w595 w685 w797 _ _] -> w455
          tunnel: [w523 w547 w573 w648 w787 w898 w978] -> w477
          tunnel: w452 -> [w539 w563 w594 _ w786 w909 w973]
          tunnel: [w539 w563 w594 w653 w788 _ _] -> w453
          tunnel: [_ _ _ _ _ FALSE TRUE] -> w485
          tunnel: [_ _ _ _ w795 _ _] -> w445
          tunnel: [_ _ _ _ w789 _ _] -> w430
          tunnel: [_ _ _ _ w794 _ _] -> w444
          tunnel: [_ _ _ _ w793 _ _] -> w443
          tunnel: [_ _ _ _ w792 _ _] -> w442
          tunnel: [_ _ _ _ w791 _ _] -> w441
          tunnel: [_ _ _ _ w790 _ _] -> w440
          tunnel: [w524 w548 w574 w645 w785 w896 w971] -> w478
          tunnel: [w538 w562 w593 w642 w783 _ _] -> w451
          tunnel: w450 -> [w538 w562 w593 _ w784 w897 w972]
          tunnel: [_ _ _ _ w782 _ _] -> w468
          tunnel: [_ _ _ _ w781 _ _] -> w467
          tunnel: [w537 w561 w585 "Initialize" ("Report Text") "Running" ("Report Text") "Wait for Init" ("Report Text") "Exit" ("Report Text")] -> w473
          tunnel: w488 -> [w537 w561 _ _ _ _ _]
          tunnel: [w521 w545 w571 w626 w769 w890 w968] -> w475
          tunnel: [w532 w559 w581 w623 w768 _ _] -> w457
          tunnel: [w531 w558 w580 w621 w766 _ _] -> w459
          tunnel: [w520 w544 w570 w620 w767 w889 w915] -> w474
          tunnel: w456 -> [w532 w559 w581 _ w770 w891 w969]
          tunnel: w458 -> [w531 w558 w580 _ w765 w887 w935]
          tunnel: [w519 w543 w569 w600 w764 FALSE FALSE] -> w470
          tunnel: [FALSE FALSE FALSE FALSE w754 FALSE FALSE] -> w425
          tunnel: [w528 w554 w578 w607 w753 w882 w965] -> w482
          tunnel: "Turn On DAQ" -> [w529 _ _ _ w729 _ _]
          tunnel: w484 -> [w527 w551 w577 w609 w752 w881 w964]
          tunnel: w484 -> [w526 w550 w576 w608 w747 w879 w926]
          tunnel: w484 -> [w528 w553 w578 w607 w753 w882 w965]
          tunnel: w484 -> [w525 w549 w575 w606 w745 w864 w949]
          tunnel: w484 -> [w524 w548 w574 w605 w744 w863 w963]
          tunnel: w484 -> [w523 w547 w573 w604 w741 w862 w962]
          tunnel: w484 -> [w522 w546 w572 w603 w740 w861 w961]
          tunnel: w484 -> [w521 w545 w571 w602 w734 w857 w960]
          tunnel: w484 -> [w520 w544 w570 w601 w730 w856 w934]
          tunnel: w469 -> [w519 w543 w569 w600 w733 _ _]
          tunnel: w464 -> [_ _ _ _ w739 _ _]
          tunnel: 0.5 ("Duty Cycle") -> [_ _ _ _ w738 _ _]
          tunnel: w462 -> [_ _ _ _ w736 _ _]
          tunnel: w461 -> [_ _ _ _ w737 _ _]
          tunnel: w460 -> [_ _ _ _ w735 _ _]
          tunnel: w428 -> [_ _ _ _ _ _ w959]
          tunnel: w426 -> [_ _ _ _ w728 w855 w958]
          frame "Wait for Init", Default {
            # "Hall Sensor"
            # "Motor TRIAC CCW"
            # "Motor TRIAC CW"
            # "Relay Controls"
            # "TRIAC Outputs"
            # "AO for ADC"
            n346 = Select(t=DAQ_States_Brass."Rename Devices", s=w529, f=DAQ_States_Brass."Wait for Init" ("States")) -> (s? t:f=w536:T24)
          }
          frame "Rename Devices" {
            # "Hall Sensor"
            # "Motor TRIAC CCW"
            # "Motor TRIAC CW"
            # "Relay Controls"
            # "TRIAC Outputs"
            n347 = case shown="\"LE\"" "HE/LE ?" {
              tunnel: ["VALEW_HE" "VALEW_LE"] -> w555
              frame "HE", Default {
              }
              frame "LE" {
              }
            }
            n348 = call "VALEW_Rename DAQmx Devices.vi"("cDAQ Name"=w555, "Error In"=w553) -> ("Error Out"=w554:errorcluster)  [unwired: 13 in]
          }
          frame "Verify Hardware" {
            n349 = call "DeviceListCheck.vi"("Device List"=string[] ["9481_1", "9435_1", "9435_2", "9401_1", "9269_1"], "Error In"=w577) -> ("Devices Present?"=w582:bool, "Report Text"=w585:string, "Error Out"=w584:errorcluster)  [unwired: 11 in]
            n350 = case shown="False" w582 {
              selector: w582 -> [w597 _]
              tunnel: w584 -> [w598 w599]
              tunnel: [w596 w599] -> w583
              frame False {
                n351 = property on="Turn On DAQ" class="Bool (strict)"(error in=w598, "Value"=w597) -> (error out=w596:errorcluster)  [unwired: 1 in, 1 out]
              }
              frame True {
              }
            }
            n352 = Select(t=DAQ_States_Brass."Initialize" ("f"), s=w582, f=DAQ_States_Brass."Wait for Init") -> (s? t:f=w588:T24)
          }
          frame "Initialize" {
            w614 = 4 items=["verify"=2, "reserve"=4, "commit"=3, "unreserve"=5, "abort"=6] ("action")
            w630 = 10123 items=["Finite Samples"=10178, "Continuous Samples"=10123, "Hardware Timed Single Point"=12522] ("sample mode")
            w633 = 4 items=["verify"=2, "reserve"=4, "commit"=3, "unreserve"=5, "abort"=6] ("action")
            w666 = 4 items=["verify"=2, "reserve"=4, "commit"=3, "unreserve"=5, "abort"=6] ("action")
            w667 = 4 items=["verify"=2, "reserve"=4, "commit"=3, "unreserve"=5, "abort"=6] ("action")
            w681 = 10123 items=["Finite Samples"=10178, "Continuous Samples"=10123, "Hardware Timed Single Point"=12522] ("sample mode")
            w689 = 0 items=["one channel for each line", "one channel for all lines"] ("line grouping")
            w694 = 0 items=["one channel for each line", "one channel for all lines"] ("line grouping")
            w697 = 0.0  # minimum value
            w698 = 5.0  # maximum value
            # "Hall Sensor"
            # "Motor TRIAC CCW"
            # "Motor TRIAC CW"
            # "Relay Controls"
            # "TRIAC Outputs"
            # "AO for ADC"
            n353 = call <vilib>:"DAQmx Create Task.vi"("auto cleanup"=TRUE, "error in"=w603) -> ("task out"=w655:refnum<k21>, "error out"=w656:errorcluster)  [unwired: 12 in]
            n354 = call <vilib>:"DAQmx Create Task.vi"("auto cleanup"=TRUE, "error in"=w602) -> ("task out"=w629:refnum<k21>, "error out"=w628:errorcluster)  [unwired: 12 in]
            n355 = call <vilib>:"DAQmx Create Task.vi"("auto cleanup"=TRUE, "error in"=w605) -> ("task out"=w663:refnum<k21>, "error out"=w664:errorcluster)  [unwired: 12 in]
            n356 = call <vilib>:"DAQmx Create Task.vi"("auto cleanup"=TRUE, "error in"=w604) -> ("task out"=w661:refnum<k21>, "error out"=w662:errorcluster)  [unwired: 12 in]
            n357 = call-poly <vilib>:"DAQmx Create Virtual Channel.vi"("task in"=w655, "counter"=tag "9401_1/ctr2", "error in"=w656) -> ("task out"=w658:refnum<k21>, "error out"=w686:errorcluster)  [unwired: 11 in]
            n358 = call-poly <vilib>:"DAQmx Create Virtual Channel.vi"("task in"=w663, "counter"=tag "9401_1/ctr0", "error in"=w664) -> ("task out"=w676:refnum<k21>, "error out"=w672:errorcluster)  [unwired: 11 in]
            n359 = call-poly <vilib>:"DAQmx Create Virtual Channel.vi"("task in"=w661, "counter"=tag "9401_1/ctr1", "error in"=w662) -> ("task out"=w675:refnum<k21>, "error out"=w674:errorcluster)  [unwired: 11 in]
            n360 = call-poly <vilib>:"DAQmx Create Virtual Channel.vi"("task in"=w629, "lines"=tag "9401_1/port0/line2", "error in"=w628) -> ("task out"=w635:refnum<k21>, "error out"=w636:errorcluster)  [unwired: 11 in]
            n361 = property class="DAQmx Channel"(reference=w658, error in=w686, "CO.Pulse.Term"=tag "/9401_1/PFI4") -> (reference out=w683:refnum<k21>, error out=w682:errorcluster)
            n362 = call-poly <vilib>:"DAQmx Create Virtual Channel.vi"("lines"=tag "9481_1/port0/line3", "error in"=w601) -> ("task out"=w621:refnum<k21>, "error out"=w620:errorcluster)  [unwired: 12 in]
            n363 = property class="DAQmx Channel"(reference=w676, error in=w672, "CI.CountEdges.Term"=tag "/9401_1/PFI0") -> (reference out=w671:refnum<k21>, error out=w670:errorcluster)
            n364 = property class="DAQmx Channel"(reference=w675, error in=w674, "CI.CountEdges.Term"=tag "/9401_1/PFI1") -> (reference out=w669:refnum<k21>, error out=w668:errorcluster)
            n365 = call-poly <vilib>:"DAQmx Create Virtual Channel.vi"("lines"=tag "9481_1/port0/line0:2", "name to assign"="Relay Outputs", "line grouping"=w694, "error in"=w608) -> ("task out"=w692:refnum<k21>, "error out"=w691:errorcluster)  [unwired: 10 in]
            n366 = call-poly <vilib>:"DAQmx Create Virtual Channel.vi"("lines"=tag "9435_1/port0/line0:2, 9435_2/port0/line0:3", "name to assign"="Outputs", "line grouping"=w689, "error in"=w609) -> ("task out"=w687:refnum<k21>, "error out"=w688:errorcluster)  [unwired: 10 in]
            n367 = call-poly <vilib>:"DAQmx Create Virtual Channel.vi"("maximum value"=w698, "minimum value"=w697, "physical channels"=tag "9269_1/ao0:2" ("lines"), "name to assign"="AO for ADC", "error in"=w606) -> ("task out"=w696:refnum<k21>, "error out"=w695:errorcluster)  [unwired: 9 in]
            n368 = call-poly <vilib>:"DAQmx Timing.vi"("task/channels in"=w635, "sample mode"=w630, "rate"=1000.0, "error in"=w636) -> ("task out"=w631:refnum<k21>, "error out"=w632:errorcluster)  [unwired: 10 in]
            n369 = call-poly <vilib>:"DAQmx Timing.vi"("task/channels in"=w683, "sample mode"=w681, "error in"=w682) -> ("task out"=w613:refnum<k21>, "error out"=w610:errorcluster)  [unwired: 11 in]
            n370 = call <vilib>:"DAQmx Control Task.vi"("task/channels in"=w671, "action"=w666, "error in"=w670) -> ("task out"=w644:refnum<k21>, "error out"=w647:errorcluster)  [unwired: 11 in]
            n371 = call <vilib>:"DAQmx Control Task.vi"("task/channels in"=w669, "action"=w667, "error in"=w668) -> ("task out"=w652:refnum<k21>, "error out"=w650:errorcluster)  [unwired: 11 in]
            n372 = call <vilib>:"DAQmx Control Task.vi"("task/channels in"=w613, "action"=w614, "error in"=w610) -> ("task out"=w612:refnum<k21>, "error out"=w611:errorcluster)  [unwired: 11 in]
            n373 = call <vilib>:"DAQmx Control Task.vi"("task/channels in"=w631, "action"=w633, "error in"=w632) -> ("task out"=w624:refnum<k21>, "error out"=w625:errorcluster)  [unwired: 11 in]
            n374 = flat-sequence {
              tunnel: w612 -> [w702]
              tunnel: w611 -> [w701]
              tunnel: w652 -> [w710]
              tunnel: [w710] -> w651
              tunnel: w650 -> [w709]
              tunnel: [w709] -> w649
              tunnel: w647 -> [w708]
              tunnel: [w708] -> w646
              tunnel: w644 -> [w707]
              tunnel: [w707] -> w643
              tunnel: w625 -> [w705]
              tunnel: w624 -> [w706]
              tunnel: [w704] -> w618
              tunnel: [w703] -> w617
              tunnel: [w702] -> w616
              tunnel: [w701] -> w615
              tunnel: [w714] -> w684
              tunnel: [w713] -> w685
              tunnel: [w724] -> w653
              tunnel: w651 -> [w723]
              tunnel: w649 -> [w722]
              tunnel: [w721] -> w648
              tunnel: w646 -> [w720]
              tunnel: [w719] -> w645
              tunnel: w643 -> [w718]
              tunnel: [w717] -> w642
              tunnel: [w716] -> w626
              tunnel: [w715] -> w623
              tunnel: w618 -> [w716]
              tunnel: w617 -> [w715]
              tunnel: w616 -> [w712]
              tunnel: w615 -> [w711]
              frame #0 {
                n375 = call <vilib>:"DAQmx Start Task.vi"("task/channels in"=w706, "error in"=w705) -> ("task out"=w703:refnum<k21>, "error out"=w704:errorcluster)  [unwired: 12 in]
              }
              frame #1 {
                n376 = call <vilib>:"DAQmx Start Task.vi"("task/channels in"=w718, "error in"=w720) -> ("task out"=w717:refnum<k21>, "error out"=w719:errorcluster)  [unwired: 12 in]
                n377 = call <vilib>:"DAQmx Start Task.vi"("task/channels in"=w723, "error in"=w722) -> ("task out"=w724:refnum<k21>, "error out"=w721:errorcluster)  [unwired: 12 in]
                n378 = call <vilib>:"DAQmx Start Task.vi"("task/channels in"=w712, "error in"=w711) -> ("task out"=w713:refnum<k21>, "error out"=w714:errorcluster)  [unwired: 12 in]
              }
            }
          }
          frame "Run" {
            # "Lid Lock Feedback"
            # "Is the task stopped?"
            # "Hall Sensor"
            # "Motor TRIAC CCW"
            # "Motor TRIAC CW"
            # "AO for ADC"
            # "Relay Controls"
            # "TRIAC Outputs"
            n379 = case shown="True" w736 {
              tunnel: w762 -> [w841 w846]
              tunnel: [w841 w845] -> w760
              tunnel: [w840 w844] -> w761
              tunnel: [w839 TRUE] -> w755
              tunnel: w740 -> [w840 w842]
              tunnel: w735 -> [w839 _]
              frame False {
              }
              frame True {
                n380 = call <vilib>:"DAQmx Stop Task.vi"("task/channels in"=w846, "error in"=w842) -> ("task out"=w845:refnum<k21>, "error out"=w844:errorcluster)  [unwired: 12 in]
              }
            }
            n381 = call-poly <vilib>:"DAQmx Read.vi"("task/channels in"=w770, "number of samples per channel"=-1, "timeout"=10.0, "error in"=w734) -> ("task out"=w768:refnum<k21>, "data"=w774:u8[], "error out"=w769:errorcluster)  [unwired: 9 in]
            n382 = Compound Arithmetic op=AND(w755, invert w736) -> (w757:bool)
            n383 = case shown="False" w757 {
              tunnel: w761 -> [w831 w835]
              tunnel: w760 -> [w832 w834]
              tunnel: [w832 w838] -> w759
              tunnel: [w831 w837] -> w758
              tunnel: w755 -> [w830 _]
              tunnel: [w830 FALSE] -> w754
              frame False {
              }
              frame True {
                n384 = call <vilib>:"DAQmx Start Task.vi"("task/channels in"=w834, "error in"=w835) -> ("task out"=w838:refnum<k21>, "error out"=w837:errorcluster)  [unwired: 12 in]
                n385 = Wait (ms)(milliseconds to wait=u32 1200) -> ()  [unwired: 1 out]
              }
            }
            n386 = Build Array("AC Power", "Mode Shift FB", "Lid Status") -> (w748:bool[])
            n387 = Build Array("Pressure", "Motor Current", "Temperature") -> (w746:dbl[])
            n388 = Search 1D Array(1D array=w774, element=u8 4) -> (index of element=w772:i32)  [unwired: 1 in]
            n389 = Equal?(x=w772, y=-1) -> (x = y?=w763:bool)
            n390 = Compound Arithmetic op=OR(w736, w737) -> (w756:bool)
            n391 = call-poly <vilib>:"DAQmx Read.vi"("task/channels in"=w728, "error in"=w752) -> ("task out"=w807:refnum<k21>, "data"=w806:bool[], "error out"=w805:errorcluster)  [unwired: 11 in]
            n392 = call-poly <vilib>:"DAQmx Write.vi"("task/channels in"=w804, "data"=w748, "error in"=w747) -> ("task out"=w803:refnum<k21>, "error out"=w799:errorcluster)  [unwired: 10 in, 1 out]
            n393 = call-poly <vilib>:"DAQmx Write.vi"("task/channels in"=w802, "data"=w746, "error in"=w745) -> ("task out"=w801:refnum<k21>, "error out"=w800:errorcluster)  [unwired: 10 in, 1 out]
            n394 = call-poly <vilib>:"DAQmx Read.vi"("task/channels in"=w784, "error in"=w744) -> ("task out"=w783:refnum<k21>, "data"=w743:u32, "error out"=w785:errorcluster)  [unwired: 11 in]
            "CW" <- w743
            n395 = call-poly <vilib>:"DAQmx Read.vi"("task/channels in"=w786, "error in"=w741) -> ("task out"=w788:refnum<k21>, "data"=w742:u32, "error out"=w787:errorcluster)  [unwired: 11 in]
            "CCW" <- w742
            n396 = case shown="True" "LL (M - A)" {
              tunnel: [w810 w820] -> w767
              tunnel: [w811 w819] -> w766
              tunnel: w765 -> [w813 w818]
              tunnel: [w809 w817] -> w764
              tunnel: w763 -> [_ w816]
              tunnel: "Lid Lock Feedback" -> [w812 _]
              tunnel: w733 -> [w809 w815]
              tunnel: w730 -> [w808 w814]
              frame False {
                n397 = call-poly <vilib>:"DAQmx Write.vi"("task/channels in"=w813, "data"=w812, "error in"=w808) -> ("task out"=w811:refnum<k21>, "error out"=w810:errorcluster)  [unwired: 10 in, 1 out]
              }
              frame True {
                # "Automatic Lid Lock feedback"
                n398 = case shown="True" w816 {
                  tunnel: w818 -> [w826 w829]
                  tunnel: [w825 w828] -> w820
                  tunnel: [w824 w829] -> w819
                  tunnel: [w823 w827] -> w817
                  tunnel: w815 -> [w822 w827]
                  tunnel: w814 -> [w821 w828]
                  frame False {
                    n399 = Not(x=w822) -> (.not. x?=w823:bool)
                    n400 = call-poly <vilib>:"DAQmx Write.vi"("task/channels in"=w826, "data"=w823, "error in"=w821) -> ("task out"=w824:refnum<k21>, "error out"=w825:errorcluster)  [unwired: 10 in, 1 out]
                  }
                  frame True {
                  }
                }
              }
            }
            n401 = Index Array(array=w806) -> (element #1=w795:bool, element #2=w789:bool, element #3=w794:bool, element #4=w793:bool, element #5=w792:bool, element #6=w791:bool, element #7=w790:bool)  [unwired: 7 in]
            n402 = call "Counts to Triac Direction.vi"("CCW ctr"=w742, "CW ctr"=w743) -> ("CW"=w781:bool, "CCW"=w782:bool)  [unwired: 8 in]
            n403 = case shown="False" w756 {
              tunnel: w759 -> [w852 w854]
              tunnel: w758 -> [w851 w853]
              tunnel: [w850 w854] -> w797
              tunnel: [w849 w853] -> w796
              tunnel: w739 -> [w848 _]
              tunnel: w738 -> [w847 _]
              frame False {
                n404 = property class="DAQmx Channel"(reference=w852, error in=w851, "CO.Pulse.Freq"=w848, "CO.Pulse.DutyCyc"=w847) -> (reference out=w850:refnum<k21>, error out=w849:errorcluster)
              }
              frame True {
              }
            }
            n405 = Select(t=DAQ_States_Brass."Run" ("States"), s=w729, f=DAQ_States_Brass."Shutdown" ("States")) -> (s? t:f=w777:T24)
          }
          frame "Shutdown" {
            w895 = 0.0
            w892 = FALSE ("element")
            # "Hall Sensor"
            # "Motor TRIAC CCW"
            # "Motor TRIAC CW"
            # "Relay Controls"
            # "TRIAC Outputs"
            # "AO for ADC"
            n406 = local read "AC Power"() -> (w880:bool)
            n407 = Build Array(w880, w892, w892) -> (w907:bool[])
            n408 = Build Array(w895, w895, w895) -> (w894:dbl[])
            n409 = call-poly <vilib>:"DAQmx Write.vi"("task/channels in"=w906, "data"=w907, "error in"=w879) -> ("task out"=w900:refnum<k21>, "error out"=w901:errorcluster)  [unwired: 10 in, 1 out]
            n410 = call-poly <vilib>:"DAQmx Write.vi"("task/channels in"=w887, "data"=FALSE, "error in"=w856) -> ("task out"=w886:refnum<k21>, "error out"=w885:errorcluster)  [unwired: 10 in, 1 out]
            n411 = call-poly <vilib>:"DAQmx Write.vi"("task/channels in"=w903, "data"=w894, "error in"=w864) -> ("task out"=w905:refnum<k21>, "error out"=w904:errorcluster)  [unwired: 10 in, 1 out]
            n412 = call "Time Delay4"("error in (no error)"=w901, "Delay Time (s)"=2.0) -> ("error out"=w899:errorcluster)  [unwired: 9 in]
            n413 = call <vilib>:"DAQmx Clear Task.vi"("task in"=w891, "error in"=w857) -> ("error out"=w890:errorcluster)  [unwired: 13 in]
            n414 = call <vilib>:"DAQmx Clear Task.vi"("task in"=w855, "error in"=w881) -> ("error out"=w912:errorcluster)  [unwired: 13 in]
            n415 = call <vilib>:"DAQmx Clear Task.vi"("task in"=w900, "error in"=w899) -> ("error out"=w878:errorcluster)  [unwired: 13 in]
            n416 = call <vilib>:"DAQmx Clear Task.vi"("task in"=w905, "error in"=w904) -> ("error out"=w871:errorcluster)  [unwired: 13 in]
            n417 = call <vilib>:"DAQmx Clear Task.vi"("task in"=w897, "error in"=w863) -> ("error out"=w896:errorcluster)  [unwired: 13 in]
            n418 = call <vilib>:"DAQmx Clear Task.vi"("task in"=w909, "error in"=w862) -> ("error out"=w898:errorcluster)  [unwired: 13 in]
            n419 = call <vilib>:"DAQmx Clear Task.vi"("task in"=w910, "error in"=w861) -> ("error out"=w860:errorcluster)  [unwired: 13 in]
            n420 = call <vilib>:"DAQmx Clear Task.vi"("task in"=w886, "error in"=w885) -> ("error out"=w889:errorcluster)  [unwired: 13 in]
            n421 = property on="Motor Current" class="Slide (strict)"(error in=w871, "Value"=2.5 ("Motor Current")) -> (error out=w869:errorcluster)  [unwired: 1 in, 1 out]
            n422 = property on="Turn On DAQ" class="Bool (strict)"(error in=w878, "Value"=FALSE ("Turn On DAQ")) -> (error out=w876:errorcluster)  [unwired: 1 in, 1 out]
            n423 = property on="Basket RPM" class="DigNum (strict)"(error in=w860, "Value"=1.0 ("Basket RPM")) -> (error out=w859:errorcluster)  [unwired: 1 in, 1 out]
            n424 = property on="Temperature" class="Slide (strict)"(error in=w869, "Value"=2.5 ("Temperature")) -> (error out=w867:errorcluster)  [unwired: 1 in, 1 out]
            n425 = property on="Mode Shift FB" class="Bool (strict)"(error in=w876, "Value"=FALSE ("Mode Shift FB")) -> (error out=w874:errorcluster)  [unwired: 1 in, 1 out]
            n426 = property on="Lid Status" class="Bool (strict)"(error in=w874, "Value"=FALSE ("Lid Status")) -> (error out=w873:errorcluster)  [unwired: 1 in, 1 out]
            n427 = property on="Pressure" class="Slide (strict)"(error in=w867, "Value"=0.0 ("Pressure")) -> (error out=w866:errorcluster)  [unwired: 1 in, 1 out]
          }
          frame "Exit" {
            w930 = FALSE ("element")
            w948 = 0.0
            n428 = local read "AC Power"() -> (w931:bool)
            n429 = Build Array(w931, w930, w930) -> (w927:bool[])
            n430 = call-poly <vilib>:"DAQmx Write.vi"("task/channels in"=w923, "data"=w927, "error in"=w926) -> ("task out"=w924:refnum<k21>, "error out"=w929:errorcluster)  [unwired: 10 in, 1 out]
            n431 = Build Array(w948, w948, w948) -> (w951:dbl[])
            n432 = call-poly <vilib>:"DAQmx Write.vi"("task/channels in"=w935, "data"=FALSE, "error in"=w934) -> ("task out"=w933:refnum<k21>, "error out"=w932:errorcluster)  [unwired: 10 in, 1 out]
            n433 = call-poly <vilib>:"DAQmx Write.vi"("task/channels in"=w950, "data"=w951, "error in"=w949) -> ("task out"=w947:refnum<k21>, "error out"=w946:errorcluster)  [unwired: 10 in, 1 out]
            n434 = call "Time Delay"("error in (no error)"=w929, "Delay Time (s)"=2.0) -> ("error out"=w925:errorcluster)  [unwired: 9 in]
            n435 = case shown="True" w959 {
              tunnel: w924 -> [_ w1011]
              tunnel: w979 -> [_ w1010]
              tunnel: [w983 w1009] -> w938
              tunnel: [w984 w1008] -> w978
              tunnel: [w980 w1007] -> w918
              tunnel: [w986 w1006] -> w921
              tunnel: [w987 w1005] -> w977
              tunnel: w973 -> [_ w1004]
              tunnel: w972 -> [_ w1003]
              tunnel: [w985 w1002] -> w971
              tunnel: w969 -> [_ w1001]
              tunnel: [w982 w1000] -> w968
              tunnel: w933 -> [_ w999]
              tunnel: [w981 w998] -> w916
              tunnel: w964 -> [w987 w997]
              tunnel: w925 -> [w986 w996]
              tunnel: w963 -> [w985 w995]
              tunnel: w962 -> [w984 w994]
              tunnel: w961 -> [w983 w993]
              tunnel: w960 -> [w982 w992]
              tunnel: w932 -> [w981 w991]
              tunnel: w958 -> [_ w990]
              tunnel: w947 -> [_ w989]
              tunnel: w946 -> [w980 w988]
              frame False {
              }
              frame True {
                # "Hall Sensor"
                # "Motor TRIAC CCW"
                # "Motor TRIAC CW"
                # "Relay Controls"
                # "TRIAC Outputs"
                # "AO for ADC"
                n436 = call <vilib>:"DAQmx Clear Task.vi"("task in"=w1001, "error in"=w992) -> ("error out"=w1000:errorcluster)  [unwired: 13 in]
                n437 = call <vilib>:"DAQmx Clear Task.vi"("task in"=w999, "error in"=w991) -> ("error out"=w998:errorcluster)  [unwired: 13 in]
                n438 = call <vilib>:"DAQmx Clear Task.vi"("task in"=w990, "error in"=w997) -> ("error out"=w1005:errorcluster)  [unwired: 13 in]
                n439 = call <vilib>:"DAQmx Clear Task.vi"("task in"=w1011, "error in"=w996) -> ("error out"=w1006:errorcluster)  [unwired: 13 in]
                n440 = call <vilib>:"DAQmx Clear Task.vi"("task in"=w989, "error in"=w988) -> ("error out"=w1007:errorcluster)  [unwired: 13 in]
                n441 = call <vilib>:"DAQmx Clear Task.vi"("task in"=w1003, "error in"=w995) -> ("error out"=w1002:errorcluster)  [unwired: 13 in]
                n442 = call <vilib>:"DAQmx Clear Task.vi"("task in"=w1004, "error in"=w994) -> ("error out"=w1008:errorcluster)  [unwired: 13 in]
                n443 = call <vilib>:"DAQmx Clear Task.vi"("task in"=w1010, "error in"=w993) -> ("error out"=w1009:errorcluster)  [unwired: 13 in]
              }
            }
            n444 = call <vilib>:"Clear Errors.vi"("error in (no error)"=w918, "specific error code to clear (0: all)"=-200088) -> ("error out"=w917:errorcluster)  [unwired: 4 in, 1 out]
            n445 = call <vilib>:"Clear Errors.vi"("error in (no error)"=w921, "specific error code to clear (0: all)"=-200088) -> ("error out"=w920:errorcluster)  [unwired: 4 in, 1 out]
            n446 = call <vilib>:"Clear Errors.vi"("error in (no error)"=w916, "specific error code to clear (0: all)"=-200088) -> ("error out"=w915:errorcluster)  [unwired: 4 in, 1 out]
            n447 = property on="Turn On DAQ" class="Bool (strict)"(error in=w920, "Value"=FALSE ("Turn On DAQ")) -> (error out=w956:errorcluster)  [unwired: 1 in, 1 out]
            n448 = property on="Motor Current" class="Slide (strict)"(error in=w917, "Value"=2.5 ("Motor Current")) -> (error out=w944:errorcluster)  [unwired: 1 in, 1 out]
            n449 = property on="Basket RPM" class="DigNum (strict)"(error in=w938, "Value"=1.0 ("Basket RPM")) -> (error out=w937:errorcluster)  [unwired: 1 in, 1 out]
            n450 = property on="Mode Shift FB" class="Bool (strict)"(error in=w956, "Value"=FALSE ("Mode Shift FB")) -> (error out=w954:errorcluster)  [unwired: 1 in, 1 out]
            n451 = property on="Temperature" class="Slide (strict)"(error in=w944, "Value"=2.5 ("Temperature")) -> (error out=w942:errorcluster)  [unwired: 1 in, 1 out]
            n452 = property on="Lid Status" class="Bool (strict)"(error in=w954, "Value"=FALSE ("Lid Status")) -> (error out=w952:errorcluster)  [unwired: 1 in, 1 out]
            n453 = property on="Pressure" class="Slide (strict)"(error in=w942, "Value"=0.0 ("Pressure")) -> (error out=w940:errorcluster)  [unwired: 1 in, 1 out]
          }
        }
        "DAQ Status" <- w473
        "DAQ On?" <- w471
        "Triac CW" <- w468
        "Traic CCW" <- w467
        "Cold Valve" <- w443
        "Recirc Pump" <- w444
        "Mode Shift" <- w430
        "Drain Pump" <- w445
        "Fabric SoftValve" <- w440
        "Spray/Rinse Valve" <- w441
        "Hot Valve" <- w442
        n454 = case shown="True" "MS (M - A)" {
          tunnel: w435 -> [w497 w508]
          tunnel: [w497 w507] -> w431
          tunnel: w430 -> [_ w498]
          frame False {
          }
          frame True {
            n455 = Equal?(x=w498, y=TRUE) -> (x = y?=w505:bool)
            n456 = case shown="True" w505 {
              tunnel: w508 -> [w513 w515]
              tunnel: [w513 w514] -> w500
              frame False {
              }
              frame True {
                n457 = Increment(x=w515) -> (x+1=w514:dbl)
              }
            }
            n458 = In Range and Coerce(upper limit=24.0, x=w500, lower limit=15.0) -> (In Range?=w502:bool)  [unwired: 1 out]
            n459 = case shown="True" w502 {
              frame False {
                n460 = property on="Mode Shift FB" class="Bool (strict)"("Value"=FALSE ("Mode Shift FB")) -> ()  [unwired: 2 in, 2 out]
              }
              frame True {
                n461 = property on="Mode Shift FB" class="Bool (strict)"("Value"=TRUE ("Mode Shift FB")) -> ()  [unwired: 2 in, 2 out]
              }
            }
            n462 = Greater Or Equal?(x=w500, y=24.0) -> (x >= y?=w499:bool)
            n463 = case shown="True" w499 {
              tunnel: w500 -> [w509 _]
              tunnel: [w509 0.0] -> w507
              frame False {
              }
              frame True {
              }
            }
          }
        }
        n464 = case shown="False" w438 {
          tunnel: w436 -> [w517 _]
          tunnel: [w516 0.0] -> w432
          frame False {
            n465 = Increment(x=w517) -> (x+1=w516:dbl)
          }
          frame True {
          }
        }
        n466 = Merge Errors(w482, w481, w480, w479, w478, w477, w476, w475, w474) -> (w483:errorcluster)
        n467 = call "Error_Control_Brass.vi"("Error In"=w483) -> ("Error Out"=w495:errorcluster)  [unwired: 14 in]
      }
      n468 = while "Periodic ERD Query Loop" {
        shift-right: [w192] -> w54
        shift-left: w81 -> [w194]
        tunnel: w71 -> [w195]
        shift-right: [w189] -> _
        shift-left: _ -> [w188]
        shift-right: [w183] -> _
        shift-left: w73 -> [w185]
        shift-right: [w178] -> _
        shift-left: _ -> [w177]
        tunnel: w69 -> [w176]
        tunnel: [w175] -> w52
        shift-right: [w174] -> _
        shift-left: _ -> [w173]
        tunnel: w65 -> [w172]
        i -> [w171]
        stop <- w191 stop-if-true
        # "ERD Loop"
        n469 = Dequeue Element(queue=w195, timeout in ms (-1)=0, error in (no error)=w194) -> (element=w180:T25, timed out?=w186:bool, error out=w193:errorcluster)  [unwired: 1 out]
        n470 = Unbundle By Name(w180) -> ("State"=w170:T26)
        n471 = Select(t=w185, s=w186, f=w170) -> (s? t:f=w184:T26)
        n472 = call "FGV_GEA2_Ref.vi"("Action"=enum16{"Set Ref", "Get Ref"}."Get Ref", "Error In"=w193) -> ("GEA2 Reference Out"=w179:refnum<k24>, "Error Out"=w182:errorcluster)  [unwired: 12 in]
        n473 = case shown="\"Read Faults\"" w184 {
          tunnel: w182 -> [w205 w213 w226 w240 w260 w300 w347 w375 w383]
          tunnel: [w197 w209 w219 w240 w258 w299 w344 w375 w383] -> w190
          tunnel: [_ _ _ _ _ _ _ _ TRUE] -> w191
          tunnel: [w204 w211 w217 w243 w264 w293 w354 w376 w381] -> w189
          tunnel: w188 -> [w204 w211 w238 w243 w264 w293 w354 w376 w381]
          tunnel: T7 {"Source"=229, "Destination"=52} ("GEA Inputs") -> [_ _ w215 _ w248 w297 _ _ _]
          tunnel: [ERD_Loop_States_Brass."Build ERD Read List" ("State") ERD_Loop_States_Brass."Read ERDs" ("State") ERD_Loop_States_Brass."Update UI" ("State") ERD_Loop_States_Brass."Update Graphs" ("State") ERD_Loop_States_Brass."Read Faults" ("State") ERD_Loop_States_Brass."Log Data" ("State") ERD_Loop_States_Brass."Read ERDs" ("State") ERD_Loop_States_Brass."Pause" ("State") ERD_Loop_States_Brass."Shutdown" ("State")] -> w183
          tunnel: w179 -> [_ _ w227 _ w253 w298 _ _ _]
          tunnel: [w202 w212 w216 w245 w262 w294 w353 w373 w379] -> w178
          tunnel: w177 -> [w202 _ w216 w245 w262 w294 w353 w373 w379]
          tunnel: w176 -> [w201 w208 w224 w241 w261 w292 w352 w372 w378]
          tunnel: [w201 w208 w224 w241 w261 w292 w351 w372 w378] -> w175
          tunnel: [w200 w207 w218 w242 w252 w295 w330 w371 w377] -> w174
          tunnel: w173 -> [w200 w207 _ w242 w250 w296 w330 w371 w377]
          tunnel: w172 -> [_ _ _ _ w254 _ _ _ _]
          tunnel: w171 -> [_ _ _ _ _ _ _ _ _]
          frame "Init", Default {
            # "Set Write Header\nFGV to True"
            n474 = call "Write_Header_FGV.vi"("Write Header ? In"=TRUE, "Action"=enum16{"Get", "Set"}."Set", "Error In"=w205) -> ("Error Out"=w197:errorcluster)  [unwired: 11 in, 1 out]
          }
          frame "Build ERD Read List" {
            n475 = call "ERD_Read_List_Builder.vi"("Array"="ERD Read List", "Error In"=w213) -> ("Read ERD List"=w212:T8[], "Error Out"=w209:errorcluster)  [unwired: 16 in]
          }
          frame "Read ERDs" {
            n476 = call "Convert Read ERD List to Message.vi"("GEA Inputs"=w215, "Read ERD List"=w216, "Error In"=w226) -> ("GEA Message"=w235:T5, "Error Out"=w236:errorcluster)  [unwired: 11 in]
            n477 = call "GEA2MessageFormatter.vi"("Prefix(Send/Recv)"="SEND", "GEA2 Data In"=w235, "Error In"=w236) -> ("Output String"=w234:string, "Error Out"=w233:errorcluster)  [unwired: 11 in]
            n478 = call "GExplorer_Queue_GEA2.vi"("Output String"=w234, "error in (no error)"=w233) -> ("error out"=w231:errorcluster)  [unwired: 13 in]
            n479 = Tick Count (ms)() -> (millisecond timer value=w217:u32)
            n480 = Subtract(x=w217, y=w238) -> (x-y=→"Log Rate (ms)":u32)
            n481 = call "GEA2 Read ERD Multiple Messages.vi"("GEA2 Reference In"=w227, "Retry Count"=1, "Read Timeout (ms)"=u32 200, "GEA Inputs"=w215, "Read ERD List"=w216, "Error In"=w231, "#ERDs per message"=7, "Verify ERD Response?"=FALSE) -> ("ERD Data Out"=w214:T34[], "Error Out"=w223:errorcluster)  [unwired: 4 in, 2 out]
            n482 = call "Write_Header_FGV.vi"("Action"=enum16{"Get", "Set"}."Get", "Error In"=w223) -> ("Write Header ? Out"=w220:bool, "Error Out"=w222:errorcluster)  [unwired: 12 in]
            n483 = call "Convert_ERDs_Brass.vi"("New Header?"=w220, "Array"=w214, "Error In"=w222) -> ("All_ERD_Data_Bundled_Brass"=w218:T35, "Error Out"=w219:errorcluster)  [unwired: 11 in]
          }
          frame "Update UI" {
            n484 = Unbundle By Name(w242) -> ("Version"=→"Version":T6, "ERD_Always Show"=→"ERD_Always Show":T1)
          }
          frame "Update Graphs" {
            n485 = case shown="True" "ERD Graphing ON" {
              tunnel: w260 -> [w281 w289]
              tunnel: [w281 w288] -> w259
              tunnel: "ERD Graph Cntrl" -> [_ w287]
              tunnel: [_ w286] -> w255
              tunnel: w253 -> [_ w285]
              tunnel: w250 -> [w280 w284]
              tunnel: [w280 w283] -> w249
              tunnel: w248 -> [_ w282]
              frame False {
              }
              frame True {
                n486 = call "Graph ERD Read List_Brass.vi"("GEA2 Reference In"=w285, "GEA Inputs"=w282, "All_Bundled_Data_Brass"=w284, "ERD Graph Cntrl"=w287, "Error In"=w289) -> ("ERD Graph  Ind"=w286:T11, "All_Bundled_Data_Brass 2"=w283:T35, "Error Out"=w288:errorcluster)  [unwired: 7 in, 1 out]
              }
            }
            n487 = case shown="True" "Graphing ON" {
              tunnel: w259 -> [w265 w279]
              tunnel: [w265 w278] -> w258
              tunnel: w255 -> [_ w276]
              tunnel: w254 -> [_ w271]
              tunnel: w249 -> [w266 w270]
              tunnel: [w266 w270] -> w252
              frame False {
              }
              frame True {
                n488 = call "Update Graphs_Brass.vi"("Select Graph"="Select Graph", "appended array"=w271, "ERD Graph  Ind 2"=w276, "All_Bundled_Data_Brass"=w270, "Error In"=w279) -> ("All Loads"=→"All Loads":u16[][], "Water Temperature"=→"Water Temperature":dbl, "Basket Speed"=→"Basket Speed":u16, "Pressure"=→"Pressure 2":dbl, "ERD 3"=→"ERD 3":dbl, "ERD 2"=→"ERD 2":dbl, "ERD 1"=→"ERD 1":dbl, "Error Out"=w278:errorcluster)  [unwired: 3 in]
                "ERD Graph  Ind" <- w276
              }
            }
          }
          frame "Read Faults" {
            n489 = case shown="True" "Fault ON" {
              tunnel: w300 -> [w301 w310]
              tunnel: [w301 w309] -> w299
              tunnel: w298 -> [_ w308]
              tunnel: w297 -> [_ w307]
              tunnel: w296 -> [w302 w306]
              tunnel: [w302 w305] -> w295
              frame False {
              }
              frame True {
                # "0-11 Sequence\n12-20 Table"
                n490 = call "GEA2 Read ERD Multiple Messages.vi"("GEA2 Reference In"=w308, "Retry Count"=2, "Read Timeout (ms)"=u32 250 ("Read Timeout (ms) 2"), "GEA Inputs"=w307, "Read ERD List"=T8[] [{"ERD Number"=132, "Data Type"=enum."string"}, {"ERD Number"=141, "Data Type"=enum."uint32_t"}, {"ERD Number"=57394, "Data Type"=enum."string"}, {"ERD Number"=57395, "Data Type"=enum."string"}, {"ERD Number"=57396, "Data Type"=enum."string"}, {"ERD Number"=57397, "Data Type"=enum."string"}, {"ERD Number"=57398, "Data Type"=enum."string"}, {"ERD Number"=57399, "Data Type"=enum."string"}, {"ERD Number"=57400, "Data Type"=enum."string"}, {"ERD Number"=57401, "Data Type"=enum."string"}, {"ERD Number"=57402, "Data Type"=enum."string"}, {"ERD Number"=57403, "Data Type"=enum."string"}, {"ERD Number"=129, "Data Type"=enum."string"}, {"ERD Number"=57444, "Data Type"=enum."string"}, {"ERD Number"=57445, "Data Type"=enum."string"}, {"ERD Number"=57446, "Data Type"=enum."string"}, {"ERD Number"=57447, "Data Type"=enum."string"}, {"ERD Number"=57448, "Data Type"=enum."string"}, {"ERD Number"=57449, "Data Type"=enum."string"}, {"ERD Number"=57450, "Data Type"=enum."string"}, {"ERD Number"=57451, "Data Type"=enum."string"}], "Error In"=w310, "#ERDs per message"=5 ("#ERDs per message 2"), "Verify ERD Response?"=FALSE) -> ("ERD Data Out"=w315:T34[], "Error Out"=w309:errorcluster)  [unwired: 4 in, 2 out]
                n491 = Array Subset(array=w315, index=12, length=11) -> (w316:T34[])
                n492 = Array Subset(array=w315, index=0, length=12) -> (w314:T34[])
                n493 = call "Fault_Table_Read.vi"("ERD Data Out"=w316) -> ("Fault Set?"=→"Fault Status":bool, "Table Buffer Status"=→"Table Buffer Status":T15, "Fault Table String Out"=→"Fault Table Buffer":string[][], "Fault Table Array Out"=w304:T37)  [unwired: 11 in]
                n494 = call "Fault_Seq_Read.vi"("Seq ERD In"=w314) -> ("Seq Buffer Status"=→"Seq Buffer Status":T15, "String"=→"Fault Sequence Buffer":string)  [unwired: 13 in]
                n495 = Bundle By Name(cluster=w306, "Fault Table Array"=w304) -> (w305:T35)
              }
            }
          }
          frame "Log Data" {
            # "TimeStamp"
            # "Append With Fault Log Data"
            # "Write Date/Time Header"
            n496 = Unbundle By Name(w330) -> ("CSV File String Arrays.ERD Name Array"=w350:string[], "CSV File String Arrays.ERD Number Array"=w349:string[], "CSV File String Arrays.ERD Converted String Data"=w342:string[])
            n497 = call "Write_Header_FGV.vi"("Action"=enum16{"Get", "Set"}."Get", "Error In"=w347) -> ("Write Header ? Out"=w328:bool, "Error Out"=w341:errorcluster)  [unwired: 12 in]
            n498 = case shown="True" w328 {
              tunnel: w350 -> [w363 _]
              tunnel: [w365 string[] [] ("ERD Name Array")] -> w340
              tunnel: w349 -> [w364 _]
              tunnel: [w368 string[] [] ("ERD Number Array")] -> w338
              frame True {
                n499 = Insert Into Array(array=w364, index=0, new element #1="", new element #2="", new element #3="", new element #4="") -> (w368:string[])
                n500 = Insert Into Array(array=w363, index=0, new element #1="Date", new element #2="Time", new element #3="HH:MM:SS", new element #4=".SS" ("new element/subarray")) -> (w365:string[])
              }
              frame False {
              }
            }
            n501 = call "TimeStamp to String Array.vi"("String Array In"=w342) -> ("String Array Out"=w336:string[])  [unwired: 10 in]
            n502 = Unbundle By Name(w330) -> ("Fault Table Array"=w329:T37)
            n503 = call "Faults_To_String_Array.vi"("Write Header ?"=w328, "Fault Table Entry"=w329, "Error In"=w341) -> ("Fault Header String Array"=w335:string[], "Fault ERD Number String Array"=w334:string[], "Fault Data String Array"=w333:string[], "Error Out"=w331:errorcluster)  [unwired: 13 in]
            n504 = Insert Into Array(array=w340, new element=w335) -> (w339:string[])  [unwired: 1 in]
            n505 = Insert Into Array(array=w338, new element=w334) -> (w337:string[])  [unwired: 1 in]
            n506 = Insert Into Array(array=w336, new element=w333) -> (w332:string[])  [unwired: 1 in]
            n507 = call "Write _To_CSV_File.vi"("Refnum In"=w352, "String Array 1"=w339, "String Array 2"=w337, "String Array 3"=w332, "Error In"=w331) -> ("Refnum Out"=w351:refnum<file>, "Error Out"=w345:errorcluster)  [unwired: 12 in, 1 out]
            n508 = call "Write_Header_FGV.vi"("Write Header ? In"=FALSE, "Action"=enum16{"Get", "Set"}."Set", "Error In"=w345) -> ("Error Out"=w344:errorcluster)  [unwired: 11 in, 1 out]
          }
          frame "Pause" {
          }
          frame "Shutdown" {
          }
        }
        n509 = call "Error_Control_Brass.vi"("Error In"=w190) -> ("Error Out"=w192:errorcluster)  [unwired: 14 in]
      }
      n510 = while "GEA2 Receive Message Loop" {
        shift-right: [w1737] -> w131
        shift-left: w37 -> [w1738]
        shift-right: [w1734] -> _
        shift-left: w120 -> [w1739]
        stop <- w1736 stop-if-true
        # "GEA2 Receive Message Loop"
        n511 = event shown="[0] <Data>: User Event" {
          selector: w1739 -> [w1755 w1757 w1773 w1779]
          dyn-events: [w1755 w1757 w1768 w1779] -> w1734
          timeout: _ -> [_ _ _ _]
          tunnel: w1738 -> [w1754 w1759 w1776 w1781]
          tunnel: [w1742 w1759 w1761 w1781] -> w1735
          tunnel: [FALSE TRUE _ TRUE] -> w1736
          event User Event {
            n512 = event-data() -> ("Source"=w1749:u8, "Destination"=w1748:u8, "Command"=w1747:u8, "Message"=w1746:string)  [unwired: 1 in]
            n513 = Bundle By Name(cluster=T5 {"Source"=0, "Destination"=0, "Command"=0, "Message"=""} ("GEA2 Msg"), "Source"=w1749, "Destination"=w1748, "Command"=w1747, "Message"=w1746) -> (w1740:T5)
            n514 = call "GEA2 Log Filter.vi"("Filter Log"="Filter Log", "Filter Data"="Filter Data", "GEA2 Msg"=w1740, "Cmd to Filter"="Cmd", "error in (no error)"=w1754) -> ("error out"=w1743:errorcluster)  [unwired: 10 in]
            n515 = call "FGV_GEA2_Ref.vi"("Action"=enum16{"Set Ref", "Get Ref"}."Get Ref", "Error In"=w1743) -> ("GEA2 Reference Out"=w1741:refnum<k24>, "Error Out"=w1744:errorcluster)  [unwired: 12 in]
            n516 = call "ACK Subscriptions Publications.vi"("GEA2 Reference In"=w1741, "GEA2 Msg"=w1740, "error in (no error)"=w1744) -> ("error out"=w1742:errorcluster)  [unwired: 11 in, 1 out]
          }
          event User Event {
            n517 = event-data() -> ()  [unwired: 1 in, 1 out]
          }
          event "Board Index": Value Change {
            # "Stop old GEA2\nbus reference"
            # "Allow other references a chance\nto begin using new reference"
            # "Store new GEA2 bus reference"
            # "Update event registration\nand initialize new GEA2 bus"
            # "Get the previous GEA2\nbus ref, but don't stop it\nuntil we update the FGV\nwith the new GEA2 ref"
            n518 = event-data() -> ("NewVal"=w1772:u8)  [unwired: 1 in]
            n519 = property on="Board Index" class="DigNum (strict)"(error in=w1776, "DisabledEnum"=T29."Disabled and Grayed Out" ("Disabled")) -> (error out=w1777:errorcluster)  [unwired: 1 in, 1 out]
            n520 = call "FGV_GEA2_Ref.vi"("Action"=enum16{"Set Ref", "Get Ref"}."Get Ref", "Error In"=w1777) -> ("GEA2 Reference Out"=w1760:refnum<k24>, "Error Out"=w1774:errorcluster)  [unwired: 12 in]
            n521 = call "GEA2_Reregister.vi"("Board Index"=w1772, "Event Registration In"=w1773, "Error In"=w1774) -> ("GEA2 Reference Out"=w1766:refnum<k24>, "Board ID"=w1769:string, "Event Registration Out"=w1768:refnum<event-registration>, "Error Out"=w1770:errorcluster)  [unwired: 9 in]
            n522 = property on="Board Index" class="DigNum (strict)"(error in=w1770, "DisabledEnum"=T29."Enabled" ("Disabled")) -> (error out=w1767:errorcluster)  [unwired: 1 in, 1 out]
            n523 = local write "Board ID"(w1769) -> ()
            n524 = call "FGV_GEA2_Ref.vi"("GEA2 Reference In"=w1766, "Action"=enum16{"Set Ref", "Get Ref"}."Set Ref", "Error In"=w1767) -> ("Error Out"=w1763:errorcluster)  [unwired: 11 in, 1 out]
            n525 = call "Time Delay"("error in (no error)"=w1763, "Delay Time (s)"=3.0) -> ("error out"=w1762:errorcluster)  [unwired: 9 in]
            n526 = call "GEA2 Stop.vi"("GEA2 Reference In"=w1760, "Error In"=w1762) -> ("Error Out"=w1761:errorcluster)  [unwired: 13 in]
          }
          event "Stop": Value Change {
            n527 = event-data() -> ()  [unwired: 1 in, 6 out]
          }
        }
        n528 = call "Error_Control_Brass.vi"("Error In"=w1735) -> ("Error Out"=w1737:errorcluster)  [unwired: 14 in]
      }
      n529 = while "Continuous Send Loop" {
        shift-right: [w145] -> _
        shift-left: Cont_Send_States."Run" ("State") -> [w144]
        tunnel: w42 -> [w146]
        tunnel: [w139] -> _
        shift-right: [w137] -> w46
        shift-left: w37 -> [w148]
        stop <- w147 stop-if-true
        # "Continuous Send Loop"
        n530 = Dequeue Element(queue=w146, timeout in ms (-1)=0, error in (no error)=w148) -> (queue out=w140:refnum<queue>, element=w133:T21, timed out?=w141:bool, error out=w136:errorcluster)
        n531 = Select(t=w144, s=w141, f=w133) -> (s? t:f=w143:T21)
        n532 = property on="GEA2 Send" class="Clust (strict)"() -> ("Value"=w135:T5)  [unwired: 2 in, 2 out]
        n533 = case shown="\"Run\", Default" w143 {
          selector: w143 -> [w152 w167]
          tunnel: w136 -> [w154 w169]
          tunnel: [w153 w169] -> w138
          tunnel: [_ TRUE] -> w147
          tunnel: [w152 w167] -> w145
          tunnel: w140 -> [w151 w166]
          tunnel: [w151 w166] -> w139
          tunnel: w135 -> [w150 _]
          frame "Run", Default {
            n534 = case shown="True" "Start Send" {
              tunnel: w154 -> [w155 w158]
              tunnel: [w155 w162] -> w153
              tunnel: w150 -> [_ w160]
              frame False {
              }
              frame True {
                n535 = call "FGV_GEA2_Ref.vi"("Action"=enum16{"Set Ref", "Get Ref"}."Get Ref", "Error In"=w158) -> ("GEA2 Reference Out"=w156:refnum<k24>, "Error Out"=w157:errorcluster)  [unwired: 12 in]
                n536 = call "GEA2MessageFormatter.vi"("Prefix(Send/Recv)"="SEND", "GEA2 Data In"=w160, "Error In"=w157) -> ("Output String"=w161:string, "Error Out"=w165:errorcluster)  [unwired: 11 in]
                n537 = call "GExplorer_Queue_GEA2.vi"("Output String"=w161, "error in (no error)"=w165) -> ("error out"=w163:errorcluster)  [unwired: 13 in]
                n538 = call "GEA2 Send Message.vi"("GEA2 Reference In"=w156, "Input Data"=w160, "Error In"=w163) -> ("Error Out"=w162:errorcluster)  [unwired: 11 in, 1 out]
              }
            }
          }
          frame "Shutdown" {
          }
        }
        n539 = call "Error_Control_Brass.vi"("Error In"=w138) -> ("Error Out"=w137:errorcluster)  [unwired: 14 in]
        n540 = Wait (ms)(milliseconds to wait="Msg Rate (ms)") -> ()  [unwired: 1 out]
      }
      n541 = while "GEA2 Display Loop" {
        tunnel: w72 -> [w393]
        shift-right: [w390] -> _
        shift-left: _ -> [w396]
        shift-right: [w392] -> w101
        shift-left: w36 -> [w400]
        tunnel: w34 -> [w386]
        tunnel: [w384] -> w32
        stop <- w394 stop-if-true
        # "GEA2 Display Loop"
        n542 = Dequeue Element(queue=w393, error in (no error)=w400) -> (element=w399:T23, error out=w395:errorcluster)  [unwired: 1 in, 2 out]
        n543 = Unbundle By Name(w399) -> ("Data"=w397:variant, "State"=w398:enum16{"Add to Log", "Clear", "Shutdown"})
        n544 = case shown="\"Add to Log\", Default" w398 {
          tunnel: w397 -> [w411 _ _]
          tunnel: w396 -> [w414 w419 _]
          tunnel: [w413 w419 ""] -> w391
          tunnel: w395 -> [w412 w420 w424]
          tunnel: [w409 w420 w424] -> w387
          tunnel: [FALSE TRUE FALSE] -> w394
          tunnel: [w401 _ _] -> w385
          frame "Add to Log", Default {
            n545 = Variant To Data(error in=w412, type="", Variant=w411) -> (data=w403:string, error out=w409:errorcluster)
            n546 = String Subset(string=w403, offset (0)=22, length (rest)=7 ("length (rest)")) -> (substring=w404:string)
            n547 = Equal?(x="SEND E5", y=w404) -> (x = y?=w402:bool)
            n548 = case shown="True" w402 {
              tunnel: w414 -> [w417 w418]
              tunnel: [w416 w418] -> w413
              tunnel: w403 -> [w415 _]
              tunnel: [w415 _] -> w401
              frame False {
                n549 = Concatenate Strings(w415, w417) -> (w416:string)
              }
              frame True {
              }
            }
          }
          frame "Shutdown" {
          }
          frame "Clear" {
          }
        }
        "GEA2 Log" <- w391
        n550 = call "Write _To_TXT_File.vi"("refnum"=w386, "text"=w385, "error in"=w387) -> ("refnum out"=w384:refnum<file>, "error out"=w388:errorcluster)  [unwired: 10 in, 1 out]
        n551 = call "Error_Control_Brass.vi"("Error In"=w388) -> ("Error Out"=w392:errorcluster)  [unwired: 14 in]
        n552 = String Subset(string=w391, length (rest)="GEA2 Log Length") -> (substring=w390:string)  [unwired: 1 in]
      }
      n553 = Close File(refnum=w32, error in=w101) -> (error out=w33:errorcluster)  [unwired: 1 out]
      n554 = call "GEA2 Stop.vi"("GEA2 Reference In"=w129, "Error In"=w130) -> ("Error Out"=w113:errorcluster)  [unwired: 13 in]
      n555 = Close File(refnum=w52, error in=w54) -> (error out=w53:errorcluster)  [unwired: 1 out]
      n556 = Merge Errors(w53, w33, w46, w131, w113, w100) -> (w28:errorcluster)
      n557 = Obtain Queue(name (unnamed)="Continuous Send", element data type=Cont_Send_States_Brass."Run" ("State"), error in (no error)=w28) -> (queue out=w51:refnum<queue>, error out=w50:errorcluster)  [unwired: 2 in, 1 out]
      n558 = Obtain Queue(name (unnamed)="ERD Loop", element data type=T25 {"Data"=variant, "State"=enum."Read ERDs"} ("Data"), error in (no error)=w28) -> (queue out=w108:refnum<queue>, error out=w107:errorcluster)  [unwired: 2 in, 1 out]
      n559 = Obtain Queue(name (unnamed)="GEA2", element data type=T23 {"Data"=variant, "State"=enum."Add to Log"} ("Data"), error in (no error)=w28) -> (queue out=w117:refnum<queue>, error out=w116:errorcluster)  [unwired: 2 in, 1 out]
      n560 = Obtain Queue(name (unnamed)="DAQ", element data type=DAQ_States_Brass."Wait for Init" ("States"), error in (no error)=w28) -> (queue out=w103:refnum<queue>, error out=w104:errorcluster)  [unwired: 2 in, 1 out]
      n561 = Release Queue(queue=w51, error in (no error)=w50) -> (error out=w49:errorcluster)  [unwired: 1 in, 2 out]
      n562 = Release Queue(queue=w108, error in (no error)=w107) -> (error out=w96:errorcluster)  [unwired: 1 in, 2 out]
      n563 = Release Queue(queue=w117, error in (no error)=w116) -> (error out=w97:errorcluster)  [unwired: 1 in, 2 out]
      n564 = Release Queue(queue=w103, error in (no error)=w104) -> (error out=w98:errorcluster)  [unwired: 1 in, 2 out]
      n565 = Merge Errors(w49, w96, w97, w98) -> (w95:errorcluster)
      n566 = call "Error_Control_Brass.vi"("Command (Handle Errors)"=Error_Command_Brass."Report Errors", "Error In"=w95) -> ("Error Out"=w88:errorcluster)  [unwired: 13 in]
    }
    frame Error {
    }
  }
  n567 = call <vilib>:"Simple Error Handler.vi"("error in (no error)"=w5) -> ("error out"=→"Error Out":errorcluster)  [unwired: 4 in, 4 out]
